vi "Spectrum Interogation routine (SIR).vi"() -> ()   [LabVIEW 2014]
doc: "This is a pretty complex VI probably best to just e-mail me if you need help"
uses:
  Subs/Global 1.vi
  <vilib>/Utility/file.llb/Read From Spreadsheet File (DBL).vi
  <vilib>/measure/mamon.llb/Waveform Peak Detection for 1 Chan.vi
  <vilib>/Utility/file.llb/Write To Spreadsheet File (DBL).vi
  <vilib>/Utility/file.llb/Read From Spreadsheet File (string).vi
  <vilib>/Utility/file.llb/Write To Spreadsheet File (I64).vi
  <vilib>/measure/NI_MAPro.lvlib
  <vilib>/Analysis/NI_AALBase.lvlib
panel:
  out "subarray":dbl[](array[numeric])
  out "Vally pos":sgl[][](array[numeric])
  out "mark":i32[](array[numeric])
  in  "System Save Data Button":bool
  out "Delimit":string
  out "intensities":sgl[][](array[numeric])
  out "First scan":sgl[][](array[numeric])
  out "Important thing L":i32[](array[numeric])
  out "Important thing R":i32[](array[numeric])
  out "Data layout":u16
  out "File style":enum32{"Radio Selection 1", "Radio Selection 2"}(ring)
  out "Crop bottom":dbl
  out "Crop top":i32
  out "Croppped wave":sgl[](array[numeric])
  out "T0":i32
  out "no' length":i32
  in  "stop":bool
  in  "Tab settings":T1(tab)
  in  "Save to file":bool
  in  "Numeric":i32=1
  in  "Type":T2(radio)=enum."Manual scan frequency"
  in  "Ring":i64(ring) items=["hh:mm:ss", "hh mm ss"]
  in  "Output":T3(radio)=enum."Use time since first scan"
  in  "Gap between files":i32=1
  in  "Start file number":i32 min=0
  in  "Filename No' format":u16(ring) items=["full #"]
  in  "End wavelength":dbl=1160.0 min=0.0 max=1039.27001953125 step=1.0
  in  "Start wavelength":dbl=512.0 min=0.0 max=1039.27001953125 step=1.0
  in  "Xcol":i32 caption="X Col" min=-1 step=1
  in  "yCol":i32=1 caption="Y Col" min=0
  in  "Peak\npointyness":sgl=0.1 caption="Pointyness" min=0 step=0.1
  in  "Vally\npointyness":sgl=0.1 min=0 step=0.1
  in  "Poly order":i32=3
  in  "Minium length":i32=10
  in  "EnH choice":u16(ring) items=["Off", "Linear best fit", "Polynomial best fit", "Moving average"]
  in  "Threshold  2":dbl=1000.0 caption="Threshold" format="%.2p"
  in  "Width 2":i32=15 caption="Width" min=3
  in  "Threshold":dbl=4000.0 format="%.2p"
  in  "Width":i32=15 min=3
  in  "Tracking \nTollerance P":i32=5
  in  "Tracking \nTollerance V":i32=5
  in  "Peaks (T/F)":bool=TRUE
  in  "Vallys (T/F)":bool
  in  "% tracking \nerror":sgl=0.5
  in  "% tracking \nerror V":sgl=0.5
  in  "Lower \nthreshold":u16
  in  "Spectrum\nMoving AV":i32=1 min=1 step=1
  in  "Cross location":dbl=765.105
  in  "Norm":bool
  in  "Substract":bool
  in  "Load sub":bool
  in  "Valid Scans":i32=619
  out "first file loc":path
  out "Detecting Peaks":bool
  out "Plotting graph":bool
  out "Scan":i32(slide)=-1 max=1036 scale=-1.0..4.0
  out "Saving Data":bool
  out "Filtering Peaks":bool caption="Finished"
  out "Load indic":bool
  in  "Load":bool
  out "Number of files":i32=620
  in  "Tab Control":T4(tab)=enum."Intensity plot"
  out "Full":T5(graph)
  in  "System Save Data Button 2":bool
  in  "Play as movie":bool
  in  "ms per scan":u32=100
  in  "Scrollbar":i32(c297)
  out "Movie Plot":T6(graph)
  out "Scan Number":i32
  in  "Combo Box":string(combo)
  out "Intensity Graph":dbl[][](graph)
  in  "Axis Settings":bool
  in  "Save Image":bool
  in  "Top":u32(colorbox)
  in  "Bottom":u32(colorbox)=16777215
  out "Mark position":dbl
  in  "Tab Control 2":enum32{"Peak position", "Peak intensity"}(tab)
  out "Peak position vs Trace number":sgl[][](graph)
  out "Peak Intensity vs Trace number":sgl[][](graph)
  out "Number of\npeaks found":i32
  in  "Tab Control 3":enum32{"Vally position", "Vally intensity"}(tab)
  in  "save av stdev":bool
  out "Vally position vs Trace number":sgl[][](graph)=[[1.0], [1.0], [1.0], [1.0], [1.0], [1.0], [1.0], [1.0], [1.0], [1.0], [1.0], [1.0], [1.0], [1.0], [1.0], [1.0], [1.0], [1.0], [1.0], [1.0], [1.0], [1.0], [1.0], [1.0], [1.0], [1.0], [1.0], [1.0], [1.0], [1.0], [1.0], [1.0], [1.0], [1.0], [1.0], [1.0], [1.0], [1.0], [1.0], [1.0], [1.0], [1.0], [1.0], [1.0], [1.0], [1.0], [1.0], [1.0], [1.0], [1.0], [1.0], [1.0], [1.0], [1.0], [1.0], [1.0], [1.0], [1.0], [1.0], [1.0], [1.0], [1.0], [1.0], [1.0], [1.0], [1.0], [1.0], [1.0], [1.0], [1.0], [1.0], [1.0], [1.0], [1.0], [1.0], [1.0], [1.0], [1.0], [1.0], [1.0], [1.0], [1.0], [1.0], [1.0], [1.0], [1.0], [1.0], [1.0], [1.0], [1.0], [1.0], [1.0], [1.0], [1.0], [1.0], [1.0], [1.0], [1.0], [1.0], [1.0], [1.0], [1.0], [1.0], [1.0], [1.0], [1.0], [1.0], [1.0], [1.0], [1.0], [1.0], [1.0], [1.0], [1.0], [1.0], [1.0], [1.0], [1.0], [1.0], [1.0], [1.0], [1.0], [1.0], [1.0], [1.0], [1.0], [1.0], [1.0], [1.0], [1.0], [1.0], [1.0], [1.0], [1.0], [1.0], [1.0], [1.0], [1.0], [1.0], [1.0], [1.0], [1.0], [1.0], [1.0], [1.0], [1.0], [1.0], [1.0], [1.0], [1.0], [1.0], [1.0], [1.0], [1.0], [1.0], [1.0], [1.0], [1.0], [1.0], [1.0], [1.0], [1.0], [1.0], [1.0], [1.0], [1.0], [1.0], [1.0], [1.0], [1.0], [1.0], [1.0], [1.0], [1.0], [1.0], [1.0], [1.0], [1.0], [1.0], [1.0], [1.0], [1.0], [1.0], [1.0], [1.0], [1.0], [1.0], [1.0], [1.0], [1.0], [1.0], [1.0], [1.0], [1.0], [1.0], [1.0], [1.0], [1.0], [1.0], [1.0], [1.0], [1.0], [1.0], [1.0], [1.0], [1.0], [1.0], [1.0], [1.0], [1.0], [1.0], [1.0], [1.0], [1.0], [1.0], [1.0], [1.0], [1.0], [1.0], [1.0], [1.0], [1.0], [1.0], [1.0], [1.0], [1.0], [1.0], [1.0], [1.0], [1.0], [1.0], [1.0], [1.0], [1.0], [1.0], [1.0], [1.0], [1.0], [1.0], [1.0], [1.0], [1.0], [1.0], [1.0], [1.0], [1.0], [1.0], [1.0], [1.0], [1.0], [1.0], [1.0], [1.0], [1.0], [1.0], [1.0], [1.0], [1.0], [1.0], [1.0], [1.0], [1.0], [1.0], [1.0], [1.0], [1.0], [1.0], [1.0], [1.0], [1.0], [1.0], [1.0], [1.0], [1.0], [1.0], [1.0], [1.0], [1.0], [1.0], [1.0], [1.0], [1.0], [1.0], [1.0], [1.0], [1.0], [1.0], [1.0], [1.0], [1.0], [1.0], [1.0], [1.0], [1.0], [1.0], [1.0], [1.0], [1.0], [1.0], [1.0], [1.0], [1.0], [1.0], [1.0], [1.0], [1.0], [1.0], [1.0], [1.0], [1.0], [1.0], [1.0], [1.0], [1.0], [1.0], [1.0], [1.0], [1.0], [1.0], [1.0], [1.0], [1.0], [1.0], [1.0], [1.0], [1.0], [1.0], [1.0], [1.0], [1.0], [1.0], [1.0], [1.0], [1.0], [1.0], [1.0], [1.0], [1.0], [1.0], [1.0], [1.0], [1.0], [1.0], [1.0], [1.0], [1.0], [1.0], [1.0], [1.0], [1.0], [1.0], [1.0], [1.0], [1.0], [1.0], [1.0], [1.0], [1.0], [1.0], [1.0], [1.0], [1.0], [1.0], [1.0], [1.0], [1.0], [1.0], [1.0], [1.0], [1.0], [1.0], [1.0], [1.0], [1.0], [1.0], [1.0], [1.0], [1.0], [1.0], [1.0], [1.0], [1.0], [1.0], [1.0], [1.0], [1.0], [1.0], [1.0], [1.0], [1.0], [1.0], [1.0], [1.0], [1.0], [1.0], [1.0], [1.0], [1.0], [1.0], [1.0], [1.0], [1.0], [1.0], [1.0], [1.0], [1.0], [1.0], [1.0], [1.0], [1.0], [1.0], [1.0], [1.0], [1.0], [1.0], [1.0], [1.0], [1.0], [1.0], [1.0], [1.0], [1.0], [1.0], [1.0], [1.0], [1.0], [1.0], [1.0], [1.0], [1.0], [1.0], [1.0], [1.0], [1.0], [1.0], [1.0], [1.0], [1.0], [1.0], [1.0], [1.0], [1.0], [1.0], [1.0], [1.0], [1.0], [1.0], [1.0], [1.0], [1.0], [1.0], [1.0], [1.0], [1.0], [1.0], [1.0], [1.0], [1.0], [1.0], [1.0], [1.0], [1.0], [1.0], [1.0], [1.0], [1.0], [1.0], [1.0], [1.0], [1.0], [1.0], [1.0], [1.0], [1.0], [1.0], [1.0], [1.0], [1.0], [1.0], [1.0], [1.0], [1.0], [1.0], [1.0], [1.0], [1.0], [1.0], [1.0], [1.0], [1.0], [1.0], [1.0], [1.0], [1.0], [1.0], [1.0], [1.0], [1.0], [1.0], [1.0]]
  in  "Average size":dbl=1.0 min=1.0 step=1.0
  out "Peak average value":dbl[](array[numeric])
  out "Vally Intensity vs Trace number":sgl[][](graph)
  out "Number of\nvallys found":i32
  out "XY Graph":cluster{i32[], "Data AVs":dbl[]}(graph)
  in  "System Start Button":bool
  in  "Slide":dbl(slide) min=597.927001953125 max=1031.6429443359375 step=0.2 scale=597.927001953125..1031.751953125
  in  "Run":bool
  in  "QUIT":bool
  # "Time stamps"
  # "seconds"
  # "Tracking config"
  # "Peaks"
  # "Vallys"
  # "Enhanced tracking"
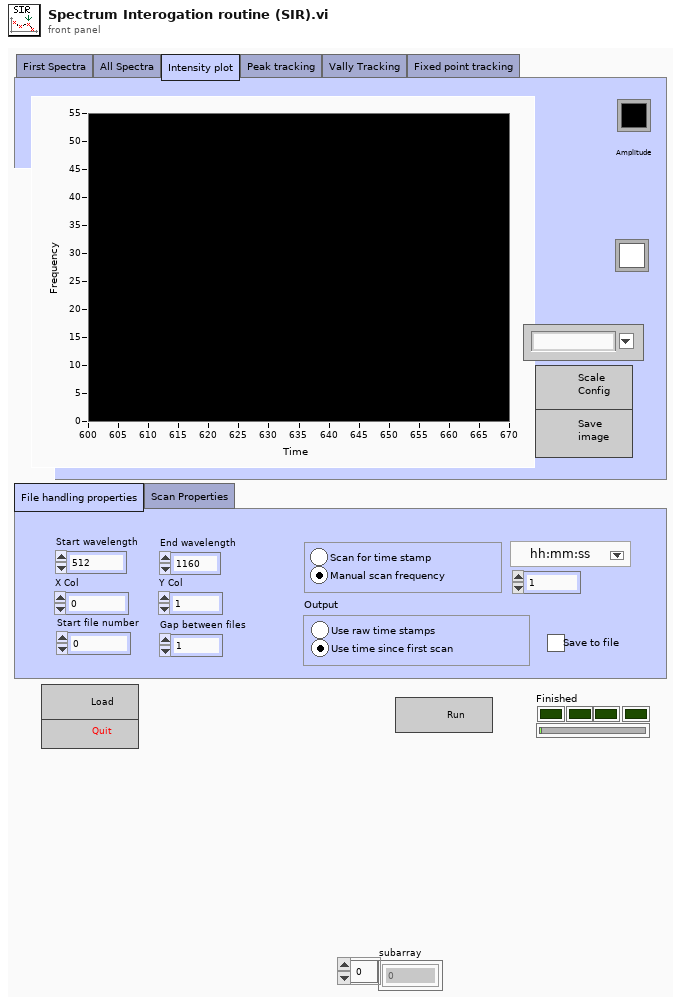
[diagram p1: front panel]
types:
  T1 = enum32{"File handling properties", "Scan Properties"}
  T2 = enum32{"Scan for time stamp", "Manual scan frequency"}
  T3 = enum32{"Use raw time stamps", "Use time since first scan"}
  T4 = enum32{"First Spectra", "All Spectra", "Intensity plot", "Peak tracking", "Vally Tracking", "Fixed point tracking"}
  T5 = cluster{"Feature locations":dbl[], "Intensities":dbl[]}[]
  T6 = cluster{"Croppped wavelengths":sgl[], "Cropped Spectrums":sgl[]}[]
  T7 = enum32{"First Spectra", "All Spectra", "Intensity plot", "Peak tracking", "Vally Tracking"}
  T8 = typedef "imagedata.ctl" = cluster{"image type":i32, "image depth":i32, "image":u8[], "mask":u8[], "colors":u32[], "Rectangle":cluster{"left":i16, "top":i16, "right":i16, "bottom":i16}}
  T9 = cluster{"YScale.Maximum":dbl, "YScale.Minimum":dbl, "YScale.ScaleFit":u8}
  T10 = cluster{"XScale.Maximum":dbl, "XScale.Minimum":dbl, "XScale.ScaleFit":u8}
  T11 = cluster{"ZScale.Maximum":dbl, "ZScale.Minimum":dbl, "ZScale.ScaleFit":u8}
  T12 = cluster{"Vally position vs Trace number":sgl[], "Vally Intensity vs Trace number":sgl[]}
  T13 = cluster{"Peak position vs Trace number":sgl[], sgl[]}
  T14 = cluster{"Croppped wave":sgl[], "intensities":sgl[]}
  T15 = cluster{"Vally position vs Trace number":sgl[], "Vally Intensity vs Trace number":sgl[]}[]
  T16 = cluster{"first file loc":path, "File style":enum32{"Radio Selection 1", "Radio Selection 2"}, "Filename No' format":u16, "Data layout":u16, "Crop top":i32, "Crop bottom":dbl, "Important thing R":i32[], "Important thing L":i32[], "First scan":sgl[][], "Delimit":string}
  T17 = cluster{"Path":path, "File style":enum32{"Radio Selection 1", "Radio Selection 2"}, "Filename No' format ":u16, "Data layout":u16, "Crop top":i32, "Crop bottom":dbl, "Important thing R":i32[], "Important thing L":i32[], sgl[][], "Delimit ":string}
  T18 = cluster{"Feature locations":dbl[], "Intensities":dbl[]}
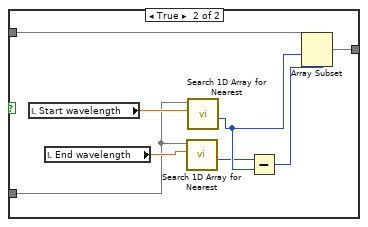
[diagram p4: hidden frame]
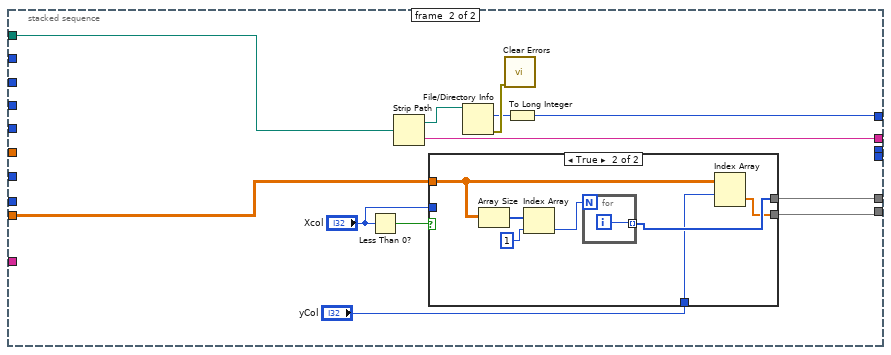
[diagram p7: hidden frame]
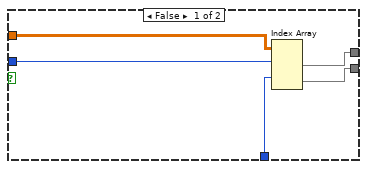
[diagram p8: hidden frame]
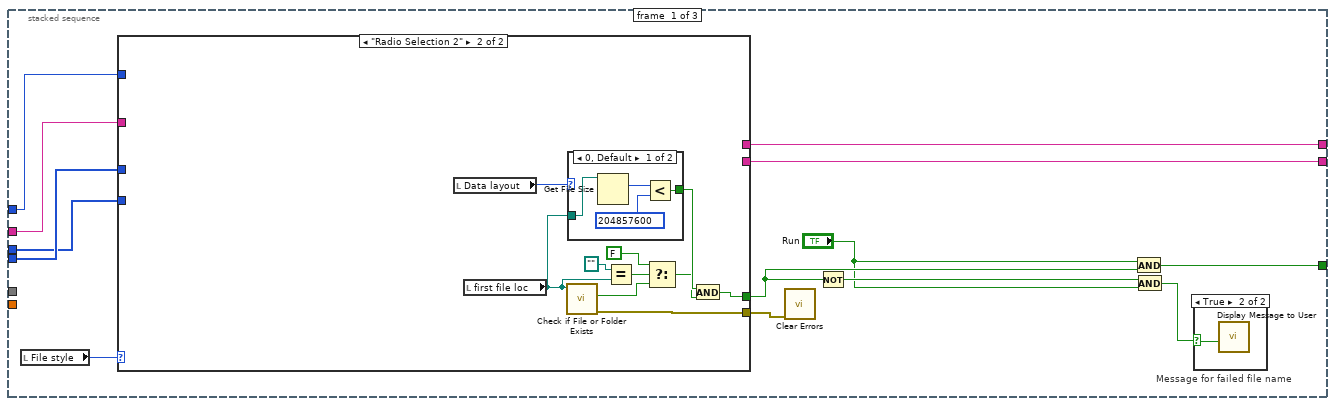
[diagram p9: hidden frame]
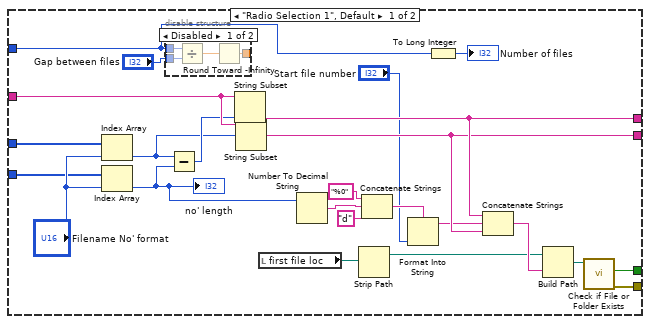
[diagram p10: hidden frame]
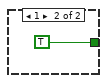
[diagram p12: hidden frame]
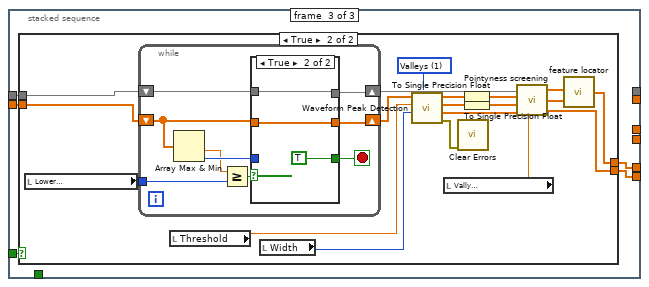
[diagram p19: hidden frame]
diagram:
  w7 = FALSE
  n1 = local write "Tab Control"(T7."First Spectra" ("Tab Control")) -> ()
  n2 = local write "First scan"(sgl[][] []) -> ()
  n3 = local write "first file loc"(path "") -> ()
  n4 = local write "QUIT"(w7) -> ()
  n5 = local write "Saving Data"(w7) -> ()
  n6 = local write "Scan"(-1) -> ()
  n7 = local write "Detecting Peaks"(w7) -> ()
  n8 = local write "Plotting graph"(w7) -> ()
  n9 = local write "Filtering Peaks"(w7) -> ()
  n10 = property on="Plotting graph" class="Bool (strict)"("Blinking"=w7) -> ()  [unwired: 2 in, 2 out]
  n11 = property on="Saving Data" class="Bool (strict)"("Blinking"=w7) -> ()  [unwired: 2 in, 2 out]
  n12 = property on="Filtering Peaks" class="Bool (strict)"("Caption.Text"="Waiting") -> ()  [unwired: 2 in, 2 out]
  n13 = property on="Filtering Peaks" class="Bool (strict)"("Blinking"=w7) -> ()  [unwired: 2 in, 2 out]
  n14 = property on="Detecting Peaks" class="Bool (strict)"("Blinking"=w7) -> ()  [unwired: 2 in, 2 out]
  n15 = local write "stop"(w7) -> ()
  n16 = property on="stop" class="Bool (strict)"("Visible"=w7) -> ()  [unwired: 2 in, 2 out]
  n17 = while {
    shift-right: [w36] -> _
    shift-left: 1 -> [w35]
    stop <- FALSE stop-if-true
    n18 = local read "EnH choice"() -> (w33:u16)
    n19 = local read "Filename No' format"() -> (w27:u16)
    n20 = Wait (ms)(milliseconds to wait=u32 10) -> ()  [unwired: 1 out]
    n21 = local read "Important thing R"() -> (w23:i32[])
    n22 = local read "Important thing L"() -> (w22:i32[])
    n23 = local read "Crop bottom"() -> (w24:dbl)
    n24 = Quit LabVIEW(quit? (T)="QUIT") -> ()
    n25 = local read "first file loc"() -> (w19:path)
    n26 = local read "Data layout"() -> (w26:u16)
    n27 = local read "Delimit"() -> (w17:string)
    n28 = local read "First scan"() -> (w21:sgl[][])
    n29 = local read "Crop top"() -> (w25:i32)
    n30 = local read "File style"() -> (w28:enum32{"Radio Selection 1", "Radio Selection 2"})
    n31 = case "Controls for individual tabs" shown="\"Intensity plot\"" "Tab Control" {
      tunnel: [w322 w324 w384 w390 w402 _] -> w36
      tunnel: w35 -> [w322 w324 w384 w390 w403 _]
      frame "First Spectra", Default {
      }
      frame "Intensity plot" {
        (unwired) u32[] [458778, 589853, 655393, 720933, 852008, 917548, 983087, 1114163, 1179703, 1310778, 1376318, 1441858, 1507397, 1572937, 1572940, 1638480, 1638484, 1704023, 1704027, 1769567, 1769570, 1769574, 1769577, 1835117, 1835121, 1835124, 1835128, 1835132, 1769599, 1769603, 1769606, 1769610, 1704078, 1704081, 1638549, 1638553, 1573020, 1573024, 1507491, 1441959, 1441963, 1376430, 1310898, 1245366, 1179834, 1114307, 1048775, 983243, 917711, 786644, 721116, 655584, 524516, 458984, 327917, 196853, 197113, 66045, 511, 1023, 264703, 528383, 792063, 792063, 1121279, 1384959, 1648639, 1912063, 2241279, 2504703, 2768383, 3031807, 3361023, 3624447, 3887871, 4151295, 4480511, 4743935, 5007359, 5270783, 5533951, 5862911, 6126335, 6389759, 6652927, 6981887, 7245055, 7508479, 7771647, 8100351, 8363775, 8626943, 8890111, 9218815, 9481983, 9745151, 10008063, 10336767, 10599935, 10863103, 11126015, 11454719, 11717631, 11980799, 12243711, 12572159, 12835071, 13098239, 13361151, 13689599, 13952511, 14215167, 14478079, 14806527, 15069439, 15332095, 15595007, 15923199, 16186111, 16448511, 16776958, 16776443, 16775671, 16775155, 16774384, 16773868, 16773096, 16772325, 16771553, 16770781, 16770010, 16769238, 16768466, 16767694, 16766923, 16766151, 16765379, 16764608, 16763580, 16762808, 16762037, 16761009, 16760237, 16759210, 16758438, 16757410, 16756382, 16755611, 16754583, 16753555, 16752528, 16751500, 16750728, 16749701, 16748673, 16747389, 16746362, 16745334, 16744306, 16743278, 16741995, 16740967, 16739939, 16738656, 16737628, 16736344, 16735061, 16734033, 16732749, 16731466, 16730438, 16729154, 16727870, 16726862, 16725835, 16724808, 16724037, 16723010, 16721984, 16721213, 16720186, 16719159, 16718389, 16717362, 16716335, 16715308, 16714538, 16713511, 16712484, 16711714, 16580642, 16580642, 16449570, 16318499, 16187427, 15859747, 15728675, 15597603, 15466531, 15269923, 15007779, 14876708, 14680100, 14549028, 14417956, 14090276, 13959204, 13828132, 13565988, 13369380, 13238308, 13041700, 12845092, 12714020, 12517412, 12320804, 12189731, 11993123, 11796515, 11665443, 11468835, 11272227, 11141155, 10944547, 10747938, 10616866, 10420258, 10223650, 10092578, 9895969, 9699361, 9568289, 9371680, 9175072, 9044000, 8847392, 8650783, 8519711, 8323103, 8126494, 7995422, 7798813, 7602205, 7471133, 7274524, 7077916, 6946843, 6750235, 6553626, 6422554, 6225945, 6029337, 5898264, 5701656, 5505047]  # Color table (Seismic)
        (unwired) u32[] [0, 257, 197379, 1285, 460551, 592137, 2571, 3085, 3599, 3857, 4114, 4628, 4886, 5144, 5402, 5660, 5918, 6176, 6434, 6691, 6693, 6951, 6953, 7211, 7213, 7471, 7473, 7475, 7477, 7478, 7480, 7482, 7484, 7486, 7232, 7491, 7236, 6980, 6469, 6213, 5957, 5702, 5446, 5191, 4935, 4424, 4168, 3912, 3657, 3145, 2890, 2634, 2123, 1867, 1612, 1100, 844, 589, 77, 78, 131150, 196687, 327759, 393295, 393295, 524368, 589904, 720977, 786513, 917586, 983122, 1114195, 1245267, 1310803, 1441876, 1572948, 1638485, 1769557, 1900630, 1966166, 2097238, 2228311, 2359383, 2424920, 2555992, 2687065, 2818137, 2949210, 3080282, 3211354, 3276891, 3473499, 3604572, 3670108, 3866717, 3997790, 4194399, 4325473, 4522082, 4718691, 4915301, 5046374, 5242983, 5439593, 5636202, 5832811, 6029421, 6291566, 6488175, 6684785, 6881394, 7143539, 7340149, 7602294, 7798903, 7929975, 7995510, 8061045, 8192116, 8257651, 8323185, 8454256, 8519791, 8585326, 8716396, 8781931, 8847466, 8978536, 9044071, 9109605, 9175139, 9306210, 9371744, 9437278, 9568349, 9633883, 9699417, 9830487, 9896021, 9961555, 10092625, 10158158, 10223692, 10354762, 10420552, 10486086, 10617156, 10682689, 10748223, 10879292, 10944826, 11010359, 11141428, 11206962, 11272495, 11403564, 11468841, 11534374, 11665443, 11730976, 11796509, 11927578, 11993111, 12189716, 12451857, 12713997, 12976138, 13303815, 13565955, 13830656, 14093824, 14356992, 14685696, 14948864, 15212032, 15344128, 15410688, 15543040, 15609600, 15741696, 15808256, 15940608, 16072961, 16140034, 16272388, 16339461, 16471815, 16538888, 16671498, 16738316, 16739597, 16740879, 16740879, 16742160, 16743442, 16744723, 16746005, 16747031, 16748312, 16749594, 16750619, 16751901, 16752926, 16753952, 16755233, 16756259, 16757285, 16758310, 16759592, 16760617, 16761643, 16762668, 16763438, 16764463, 16765489, 16766515, 16767541, 16768568, 16769597, 16770626, 16771656, 16772429, 16773458, 16774232, 16775005, 16775778, 16776295, 16777069, 16711538, 16514935, 16383868, 16252802, 16187271, 16056204, 15990673, 15925143, 15859612, 15794081, 15728551, 15728556, 15728561, 15728566, 15728572, 15728577, 15728582, 15794123, 15859665, 15925206, 15990747, 16056288, 16187366, 16252907, 16383984, 16515062, 16646139, 11184809]  # Color table (Space)
        (unwired) u32[] [16777215, 16777213, 16711675, 16646137, 16646135, 16580597, 16580595, 16515057, 16515055, 16449517, 16449515, 16449513, 16449511, 16449509, 16449507, 16449505, 16449503, 16449501, 16449499, 16449497, 16515031, 16515029, 16515027, 16580561, 16646095, 16646093, 16711627, 16777161, 16777159, 16777157, 16776899, 16776641, 16776383, 16776125, 16775867, 16775353, 16775095, 16774837, 16774323, 16774065, 16773551, 16773293, 16772778, 16772264, 16772006, 16771492, 16770978, 16770464, 16769950, 16769436, 16768922, 16768152, 16767638, 16767124, 16766610, 16765840, 16765326, 16764556, 16763786, 16763272, 16762502, 16761732, 16760962, 16760448, 16760448, 16759678, 16758908, 16757882, 16757112, 16756342, 16755572, 16754802, 16753776, 16753006, 16751980, 16751210, 16750184, 16749158, 16748388, 16747362, 16746336, 16745310, 16744284, 16743258, 16742232, 16741206, 16739923, 16738897, 16737871, 16736589, 16735563, 16734281, 16733255, 16731973, 16730691, 16729665, 16728127, 16727612, 16726592, 16726337, 16725827, 16725317, 16724807, 16724297, 16723788, 16723278, 16722768, 16722259, 16721749, 16721240, 16720731, 16720222, 16719713, 16719203, 16718695, 16718186, 16717677, 16717168, 16716660, 16716151, 16715643, 16715134, 16714626, 16714118, 16713609, 16713101, 16712593, 16712086, 16646298, 16515229, 16384161, 16253092, 16122024, 15990955, 15859887, 15728818, 15597749, 15466680, 15335611, 15204542, 15073473, 14942404, 14811334, 14680265, 14549195, 14418126, 14287056, 14155986, 14024917, 13697236, 13304018, 12910800, 12517582, 12124364, 11731146, 11337928, 11010246, 10617028, 10289346, 9896128, 9568446, 9240764, 8913082, 8585400, 8257718, 7930036, 7602354, 7274672, 6946990, 6684844, 6357162, 6095015, 5767333, 5505187, 5243041, 4980895, 4718749, 4456603, 4194457, 3932311, 3670165, 3473555, 3211409, 3014799, 2752653, 2556043, 2359433, 2162823, 1900677, 1704067, 1507457, 1376383, 1376383, 1179773, 983163, 786553, 852087, 458869, 327795, 196721, 65647, 109, 875, 1385, 1639, 2149, 3427, 3169, 3423, 3933, 4187, 4697, 4951, 5205, 5458, 5712, 5966, 6220, 6474, 6728, 6726, 6980, 6978, 7232, 7230, 7228, 7482, 7480, 7478, 7476, 7474, 7216, 7214, 7212, 6954, 6952, 6694, 6436, 6434, 6176, 5918, 5660, 5402, 5144, 4630, 4372, 4114, 3600, 3342, 2828, 2317, 2056, 1542, 1027, 131072, 0]  # Color table (Saturn)
        (unwired) u32[] [3538998, 3801146, 4128830, 4390978, 4587590, 4784201, 5046349, 5242960, 5439571, 5701719, 5898330, 6094941, 6357089, 6553700, 6815848, 7012459, 7209070, 7471218, 7667829, 7864440, 8126588, 8323199, 8519807, 8716415, 8978559, 9175167, 9371775, 9568383, 9764991, 10027135, 10223743, 10420351, 10616959, 10813567, 11010175, 11272319, 11468927, 11665535, 11862143, 12058751, 12320895, 12517503, 12714111, 12910719, 13107327, 13369471, 13566079, 13762687, 13959295, 14155903, 14352511, 14614655, 14811263, 15007871, 15204479, 15401087, 15663231, 15859839, 16056447, 16253055, 16449663, 16711807, 16712578, 16713349, 16713349, 16714121, 16714892, 16715663, 16716690, 16717461, 16718233, 16719004, 16719775, 16720802, 16721573, 16722344, 16723116, 16723887, 16724914, 16725685, 16726456, 16727228, 16727999, 16728770, 16729797, 16730568, 16731340, 16732111, 16732882, 16733909, 16734680, 16735451, 16736223, 16736994, 16738021, 16738792, 16739563, 16740335, 16741106, 16741877, 16742904, 16743675, 16744447, 16744703, 16744959, 16744959, 16745215, 16745471, 16745727, 16745983, 16746239, 16746239, 16746495, 16746751, 16747007, 16747263, 16747519, 16747519, 16747775, 16748031, 16748287, 16748543, 16748799, 16748799, 16749055, 16749311, 16749567, 16749823, 16750079, 16750079, 16750335, 16750591, 16750847, 16751103, 16751103, 16751359, 16751615, 16751871, 16752127, 16752383, 16752383, 16752639, 16752895, 16753151, 16753407, 16753663, 16753663, 16753919, 16754175, 16754431, 16754687, 16754943, 16754943, 16755199, 16755455, 16755711, 16755967, 16756223, 16756223, 16756479, 16756735, 16756991, 16757247, 16757503, 16757503, 16757759, 16758015, 16758271, 16758527, 16758527, 16758783, 16759039, 16759295, 16759551, 16759807, 16759807, 16760063, 16760319, 16760575, 16760831, 16761087, 16761087, 16761343, 16761599, 16761855, 16762111, 16762367, 16762367, 16762623, 16762879, 16763135, 16763391, 16763391, 16763647, 16763647, 16763903, 16764159, 16764415, 16764671, 16764671, 16764927, 16765183, 16765439, 16765695, 16765951, 16765951, 16766207, 16766463, 16766719, 16766975, 16767231, 16767231, 16767487, 16767743, 16767999, 16768255, 16768511, 16768511, 16768767, 16769023, 16769279, 16769535, 16769791, 16769791, 16770047, 16770303, 16770559, 16770815, 16770815, 16771071, 16771327, 16771583, 16771839, 16772095, 16772095, 16772351, 16772607, 16772863, 16773119, 16773375, 16773375, 16773631, 16773887, 16774143, 16774399, 16774655, 16774655, 16774911, 16775167, 16775423, 16775679, 16775935, 16775935, 16776191, 16776447, 16776703]  # Color table (Rose)
        (unwired) u32[] [162896, 227667, 292437, 357208, 421979, 487005, 551776, 616547, 877926, 746089, 811115, 875886, 940657, 1070964, 1135991, 1200761, 1265532, 1330303, 1395330, 1460100, 1524871, 1589898, 1654668, 1719439, 1784465, 1849236, 1914262, 1979033, 2109595, 2174366, 2239136, 2304162, 2369189, 2433959, 2498985, 2563755, 2628781, 2693807, 2758577, 2823603, 2888629, 2953654, 3018424, 3148985, 3214779, 3279036, 3344062, 3409087, 3474112, 3539138, 3604931, 3670980, 3737029, 3803077, 3869126, 3935687, 4000967, 4132552, 4198600, 4264393, 4330441, 4396233, 4462281, 4528074, 4528074, 4594121, 4659913, 4725961, 4791753, 4857544, 4923592, 4989383, 5055175, 5186502, 5252293, 5318085, 5383876, 5449667, 5515458, 5581248, 5647039, 5712830, 5778364, 5844155, 5909945, 5975480, 6041270, 6107061, 6238131, 6303665, 6369455, 6434989, 6500779, 6566313, 6631847, 6697381, 6762914, 6828448, 6893982, 6959515, 7025049, 7090582, 7221652, 7287185, 7352719, 7418252, 7483530, 7549063, 7614340, 7679874, 7745407, 7810684, 7875961, 7941495, 8006772, 8072049, 8137582, 8268395, 8333673, 8398950, 8464227, 8529504, 8594781, 8660059, 8725336, 8790613, 8855891, 8920912, 8986189, 9051466, 9116744, 9181765, 9312579, 9377600, 9442878, 9507899, 9573177, 9638198, 9703220, 9768498, 9833520, 9899310, 9963563, 10028841, 10093863, 10158885, 10223907, 10354722, 10420768, 10486814, 10552861, 10618907, 10685721, 10751000, 10817303, 10883349, 10949396, 11015443, 11081746, 11147793, 11213840, 11345679, 11411727, 11477774, 11544077, 11610125, 11676428, 11742476, 11808780, 11874828, 11941132, 12007180, 12073484, 12139788, 12205836, 12272140, 12403981, 12470029, 12536334, 12602638, 12668687, 12734992, 12801297, 12867602, 12933651, 12999956, 13066261, 13132566, 13198616, 13264921, 13331226, 13463068, 13463068, 13529374, 13595423, 13661729, 13728035, 13794341, 13860647, 13926953, 13993003, 14059309, 14125615, 14191921, 14258227, 14324278, 14456120, 14522426, 14588733, 14655039, 14721090, 14787396, 14853703, 14920010, 14986060, 15052367, 15118674, 15184980, 15251031, 15317338, 15383645, 15515231, 15581538, 15647589, 15713896, 15780202, 15846253, 15912560, 15978611, 16044918, 16110968, 16177275, 16243326, 16309377, 16375683, 16441734, 16573577, 16639627, 16705678, 16771729, 16706963, 16641942, 16576920, 16511899, 16446877, 16381855, 16316834, 16251812, 16186790, 16121768, 15990186, 15924140, 15858094, 15792048, 15726002, 15660212]  # Color table (Morning glory)
        (unwired) u32[] [3355443, 2697513, 1842204, 921102, 328965, 131586, 460551, 1184274, 2171169, 3223857, 3947580, 4276545, 4079166, 3421236, 2565927, 1644825, 1052688, 855309, 1184274, 1907997, 2894892, 3947580, 4671303, 5000268, 4802889, 4144959, 3289650, 2368548, 1776411, 1579032, 1842204, 2631720, 3618615, 4671303, 5395026, 5723991, 5526612, 4934475, 4013373, 3092271, 2500134, 2302755, 2565927, 3355443, 4342338, 5395026, 6118749, 6447714, 6250335, 5592405, 4737096, 3815994, 3223857, 3026478, 3289650, 4079166, 5066061, 6118749, 6842472, 7171437, 6974058, 6316128, 5460819, 4539717, 4539717, 3947580, 3750201, 4013373, 4802889, 5789784, 6842472, 7566195, 7895160, 7697781, 7039851, 6184542, 5263440, 4671303, 4473924, 4737096, 5526612, 6513507, 7566195, 8289918, 8618883, 8421504, 7763574, 6908265, 5987163, 5395026, 5197647, 5460819, 6250335, 7237230, 8289918, 9013641, 9342606, 9145227, 8487297, 7631988, 6710886, 6118749, 5921370, 6184542, 6974058, 7960953, 9013641, 9737364, 10066329, 9868950, 9211020, 8355711, 7434609, 6842472, 6579300, 6908265, 7697781, 8684676, 9671571, 10461087, 10790052, 10592673, 9934743, 9079434, 8158332, 7500402, 7303023, 7631988, 8421504, 9408399, 10395294, 11184810, 11513775, 11316396, 10658466, 9803157, 8882055, 8224125, 8026746, 8355711, 9145227, 10132122, 11119017, 11908533, 12237498, 12040119, 11382189, 10526880, 9605778, 8947848, 8750469, 9079434, 9868950, 10855845, 11842740, 12632256, 12961221, 12763842, 12105912, 11250603, 10329501, 9671571, 9474192, 9803157, 10592673, 11579568, 12566463, 13355979, 13684944, 13487565, 12829635, 11974326, 11053224, 10395294, 10197915, 10526880, 11316396, 12303291, 13290186, 14079702, 14408667, 14211288, 13553358, 12632256, 11776947, 11119017, 10921638, 11250603, 11974326, 13027014, 14013909, 14803425, 14803425, 15132390, 14935011, 14277081, 13355979, 12500670, 11842740, 11645361, 11974326, 12698049, 13750737, 14737632, 15527148, 15856113, 15658734, 15000804, 14079702, 13224393, 12566463, 12369084, 12698049, 13421772, 14474460, 15461355, 16250871, 16579836, 16382457, 15724527, 14803425, 13948116, 13290186, 13092807, 13421772, 14145495, 15198183, 16185078, 16645629, 16316664, 16514043, 16448250, 15527148, 14671839, 14013909, 13816530, 14145495, 14869218, 15921906, 16711422, 15921906, 15592941, 15790320, 16448250, 16250871, 15395562, 14737632, 14540253, 14869218, 15592941, 16645629, 15987699, 15198183, 14935011, 15066597, 15724527]  # Color table (GrayScale-banded)
        n32 = case "Exports intensity graph as image" shown="True" "Save Image" {
          frame False {
          }
          frame True {
            n33 = invoke on="Intensity Graph" class="IntGraph (strict)" method="Get Image"("image depth"=24 ("Image Depth")) -> (error out=w372:errorcluster, "image data"=w373:T8)  [unwired: 5 in, 4 out]
            n34 = local write "Save Image"(FALSE) -> ()
            n35 = call "File Dialog2"() -> ("selected path"=w374:path, "error out"=w371:errorcluster)  [unwired: 12 in, 2 out]
            n36 = call <vilib>:"Clear Errors.vi"("error in (no error)"=w372) -> ()  [unwired: 5 in, 2 out]
            n37 = case shown="No Error" w371 {
              tunnel: w374 -> [w382 _]
              tunnel: w373 -> [w376 _]
              frame No Error {
                n38 = Strip Path(path=w382) -> (stripped path=w378:path, name=w380:string)
                n39 = Concatenate Strings(w380, ".jpg") -> (w379:string)
                n40 = Build Path(base path=w378, name or relative path=w379) -> (appended path=w377:path)
                n41 = call <vilib>:"Write JPEG File.vi"("quality (80)"=100, "image data"=w376, "path to JPEG file"=w377) -> ()  [unwired: 7 in, 2 out]
              }
              frame Error {
              }
            }
          }
        }
        n42 = case shown="True" "Axis Settings" {
          tunnel: w324 -> [_ _]
          frame False {
          }
          frame True {
            n43 = stacked-sequence {
              tunnel: [_ w362 _] -> w342
              tunnel: [w358 _ _] -> w343
              tunnel: [_ _ w366] -> w341
              frame #0 {
                n44 = property on="Intensity Graph" class="IntGraph (strict)"() -> ("YScale.Maximum"=w361:dbl, "YScale.Minimum"=w360:dbl, "YScale.ScaleFit"=w359:u8)  [unwired: 2 in, 2 out]
                n45 = Bundle("YScale.Maximum"=w361, "YScale.Minimum"=w360, "YScale.ScaleFit"=w359) -> (w358:T9)  [unwired: 1 in]
              }
              frame #1 {
                n46 = property on="Intensity Graph" class="IntGraph (strict)"() -> ("XScale.Maximum"=w365:dbl, "XScale.Minimum"=w364:dbl, "XScale.ScaleFit"=w363:u8)  [unwired: 2 in, 2 out]
                n47 = Bundle("XScale.Maximum"=w365, "XScale.Minimum"=w364, "XScale.ScaleFit"=w363) -> (w362:T10)  [unwired: 1 in]
              }
              frame #2 {
                n48 = property on="Intensity Graph" class="IntGraph (strict)"() -> ("ZScale.Maximum"=w369:dbl, "ZScale.Minimum"=w368:dbl, "ZScale.ScaleFit"=w367:u8)  [unwired: 2 in, 2 out]
                n49 = Bundle("ZScale.Maximum"=w369, "ZScale.Minimum"=w368, "ZScale.ScaleFit"=w367) -> (w366:T11)  [unwired: 1 in]
              }
            }
            n50 = local write "Axis Settings"(FALSE) -> ()
            n51 = call "3d axis settings.vi"("Int Current"=w341, "Wave Current"=w342, "Scan Current"=w343) -> ("Int setting"=w339:T11, "Wave setting"=w340:T11, "Scan setting"=w344:T11)
            n52 = stacked-sequence {
              tunnel: w339 -> [_ _ w355]
              tunnel: w344 -> [w346 _ _]
              tunnel: w340 -> [_ w351 _]
              frame #0 {
                n53 = Unbundle(w346) -> ("ZScale.Maximum"=w349:dbl, "ZScale.Minimum"=w348:dbl, "ZScale.ScaleFit"=w347:u8)
                n54 = property on="Intensity Graph" class="IntGraph (strict)"("YScale.Maximum"=w349, "YScale.Minimum"=w348, "YScale.ScaleFit"=w347) -> ()  [unwired: 2 in, 2 out]
              }
              frame #1 {
                n55 = Unbundle(w351) -> ("ZScale.Maximum"=w353:dbl, "ZScale.Minimum"=w350:dbl, "ZScale.ScaleFit"=w352:u8)
                n56 = property on="Intensity Graph" class="IntGraph (strict)"("XScale.Maximum"=w353, "XScale.Minimum"=w350, "XScale.ScaleFit"=w352) -> ()  [unwired: 2 in, 2 out]
              }
              frame #2 {
                n57 = Unbundle(w355) -> ("ZScale.Maximum"=w357:dbl, "ZScale.Minimum"=w354:dbl, "ZScale.ScaleFit"=w356:u8)
                n58 = property on="Intensity Graph" class="IntGraph (strict)"("ZScale.Maximum"=w357, "ZScale.Minimum"=w354, "ZScale.ScaleFit"=w356) -> ()  [unwired: 2 in, 2 out]
              }
            }
          }
        }
        n59 = case shown="\"Carnation\"" "Combo Box" {
          frame "Carnation" {
            w327 = u32[] [16711691, 16711954, 16712217, 16712480, 16712742, 16713005, 16713268, 16713530, 16713793, 16714056, 16715086, 16714580, 16714842, 16715104, 16715367, 16715629, 16715891, 16716153, 16716415, 16716677, 16716940, 16717202, 16717463, 16717725, 16717987, 16718249, 16718511, 16718772, 16719034, 16719296, 16719557, 16719819, 16720079, 16720341, 16720602, 16720863, 16721125, 16721386, 16721647, 16721908, 16722169, 16722430, 16395007, 16133119, 15805695, 15478271, 15216383, 14888959, 14561535, 14234111, 13972223, 13644799, 13382911, 13055487, 12793599, 12531711, 12269823, 11942399, 11680511, 11418623, 11156735, 10829311, 10567423, 10305535, 10305535, 10043647, 9781503, 9585151, 9323263, 9061375, 8799487, 8537599, 8341247, 8079359, 7883007, 7621119, 7424767, 7228415, 6966527, 6770175, 6573823, 6377471, 6115583, 5919231, 5722879, 5526527, 5527551, 5594111, 5660927, 5727743, 5794559, 5861375, 5927935, 5994751, 6061567, 6128127, 6194943, 6261503, 6328063, 6394879, 6461439, 6527999, 6594815, 6661375, 6727935, 6794495, 6861055, 6927871, 6994175, 7060735, 7127295, 7193855, 7260415, 7326719, 7393279, 7459839, 7526143, 7592703, 7659007, 7725311, 7791871, 7858175, 7924479, 7991039, 8057343, 8123647, 8189951, 8256255, 8322815, 8388605, 8454139, 8519672, 8585205, 8650738, 8716271, 8781804, 8847338, 8912871, 8978404, 9043938, 9109472, 9175005, 9240539, 9306073, 9371606, 9437140, 9502674, 9568208, 9633742, 9699275, 9764809, 9830343, 9895877, 9961412, 10026946, 10092480, 10158014, 10223548, 10289083, 10354617, 10420152, 10485686, 10551221, 10616755, 10682290, 10747825, 10813359, 10878894, 10944429, 11009964, 11075499, 11141034, 11206570, 11403179, 11599788, 11796397, 11993006, 12124079, 12320688, 12517297, 12648370, 12844979, 13041588, 13172661, 13303734, 13500343, 13631416, 13762489, 13959098, 14090171, 14221244, 14352317, 14352317, 14483390, 14614463, 14745535, 14876608, 15007681, 15138754, 15269827, 15335364, 15466437, 15597510, 15663047, 15794120, 15859657, 15990730, 16056267, 16121804, 16252877, 16318414, 16383951, 16515024, 16580561, 16646098, 16711635, 16776916, 16776917, 16776662, 16776407, 16776152, 16775897, 16775642, 16775643, 16775388, 16775133, 16775134, 16775135, 16774880, 16774881, 16774626, 16774627, 16774628, 16774373, 16774374, 16774375, 16774376, 16774377, 16774378, 16774379, 16774380, 16774381, 16774638, 16774639, 16774640, 16774641, 16774898, 16774899, 16775156, 16775157, 16775414, 16775415, 16775672, 16775929, 16776186, 16776187]  # Color table (Carnation)
            n60 = property on="Intensity Graph" class="IntGraph (strict)"("Color Table"=w327) -> ()  [unwired: 2 in, 2 out]
          }
          frame "Hot metal" {
            w328 = u32[] [3407872, 131072, 196608, 327680, 458752, 589824, 655360, 786432, 917504, 1048576, 1114112, 1245184, 1376256, 1507328, 1572864, 1703936, 1835008, 1966080, 2031616, 2162688, 2293760, 2424832, 2555904, 2621440, 2752512, 2883584, 3014656, 3080192, 3211264, 3342336, 3473408, 3538944, 3670016, 3801088, 3932160, 3997696, 4128768, 4259840, 4390912, 4456448, 4587520, 4718592, 4849664, 4980736, 5046272, 5177344, 5308416, 5439488, 5505024, 5636096, 5767168, 5898240, 5963776, 6094848, 6225920, 6356992, 6422528, 6553600, 6684672, 6815744, 6881280, 7012352, 7143424, 7143424, 7274496, 7405568, 7471104, 7602176, 7733248, 7864320, 7929856, 8060928, 8192000, 8323072, 8388608, 8519680, 8650752, 8781824, 8847360, 8978432, 9109504, 9240576, 9306112, 9437184, 9568256, 9699328, 9830400, 9895936, 10027008, 10158080, 10289152, 10354688, 10485760, 10616832, 10747904, 10813440, 10944512, 11075584, 11206656, 11272192, 11403264, 11534336, 11665408, 11730944, 11862016, 11993088, 12124160, 12189696, 12320768, 12451840, 12582912, 12713984, 12779520, 12910592, 13041664, 13172736, 13238272, 13369344, 13500416, 13631488, 13697024, 13828096, 13959168, 14090240, 14155776, 14286848, 14417920, 14548992, 14614528, 14745600, 14876672, 15007744, 15138816, 15204352, 15335424, 15466496, 15597568, 15663104, 15794176, 15925248, 16056320, 16121856, 16252928, 16384000, 16515072, 16580608, 16580608, 16580608, 16515072, 16711680, 16711680, 16711680, 16712192, 16647424, 16713728, 16714496, 16715264, 16716032, 16716800, 16717568, 16718336, 16719104, 16719872, 16720640, 16721408, 16722176, 16722944, 16723712, 16724480, 16725248, 16726016, 16726784, 16727552, 16728064, 16728832, 16729600, 16730368, 16731136, 16731904, 16732672, 16733440, 16734208, 16734976, 16735744, 16736512, 16737280, 16738048, 16738816, 16739584, 16740352, 16741120, 16741120, 16741888, 16742656, 16743424, 16743936, 16744704, 16745472, 16746240, 16747008, 16747776, 16748544, 16749312, 16750080, 16750848, 16751616, 16752384, 16753152, 16753920, 16754688, 16755456, 16756224, 16756992, 16757760, 16758528, 16759296, 16760064, 16760576, 16761344, 16762112, 16762880, 16763648, 16764416, 16765184, 16765952, 16766720, 16767488, 16768256, 16769024, 16769792, 16770560, 16771328, 16772096, 16772864, 16773632, 16774400, 16775168, 16775936, 16776448, 16776960, 16776960, 16776960, 16776960, 16776960, 16776960, 16776960, 16776960, 16776960, 16776960, 16776960, 16776960, 16776960, 16776960, 16776960, 16776448]  # Color table (Hot metal)
            n61 = property on="Intensity Graph" class="IntGraph (strict)"("Color Table"=w328) -> ()  [unwired: 2 in, 2 out]
          }
          frame "Rainbow-striped" {
            w329 = u32[] [12255418, 12386492, 12517567, 12320960, 12189888, 12058817, 11927746, 11731139, 11600067, 9175197, 9044125, 11141318, 11010246, 10813639, 10682568, 10551497, 10354890, 10223818, 10092747, 7930019, 7798948, 9633997, 9502926, 9306319, 9175248, 9044176, 8847569, 8716498, 8585427, 6750377, 6619306, 8126677, 7995606, 7798999, 7667927, 7536856, 7340249, 7209178, 7078106, 5505199, 5374128, 6619357, 6488285, 6291678, 6160607, 6029536, 5832929, 5701857, 5570786, 4325557, 4194486, 5112036, 4980965, 4784358, 4653287, 4522215, 4325608, 4194537, 4063466, 3080380, 3014844, 3604716, 3408109, 3277038, 3277038, 3145966, 3014895, 2818288, 2687217, 2556145, 1900738, 1769666, 2097396, 1900789, 1769717, 1638646, 1507575, 1310968, 1179896, 1048825, 721096, 590024, 590075, 393468, 262397, 131326, 255, 1791, 3327, 4863, 5068, 6348, 9471, 11007, 12543, 14079, 15615, 17151, 18687, 20223, 17612, 18636, 25087, 26623, 28159, 29695, 31231, 32767, 34303, 35839, 29900, 31180, 40447, 41983, 43775, 45311, 46847, 48383, 49919, 51455, 42444, 43724, 56063, 57599, 59135, 60671, 62207, 63743, 65535, 65528, 52418, 52413, 65510, 65504, 65498, 65492, 65486, 65480, 65474, 65468, 52369, 52364, 65449, 65443, 65437, 65431, 65425, 65419, 65413, 65407, 52321, 52316, 65389, 65383, 65377, 65371, 65364, 65358, 65352, 65346, 52272, 52267, 65328, 65322, 65316, 65310, 65304, 65298, 65292, 65286, 52224, 314368, 851712, 1244928, 1638144, 2031360, 2424576, 2817792, 3211008, 3604224, 3197952, 3525632, 4783872, 5177088, 5635840, 6029056, 6422272, 6815488, 7208704, 7601920, 6409216, 6736896, 6736896, 8781568, 9174784, 9568000, 9961216, 10354432, 10747648, 11206400, 11599616, 9554944, 9882624, 12779264, 13172480, 13565696, 13958912, 14352128, 14745344, 15138560, 15531776, 12766208, 13093888, 16776960, 16775170, 16773637, 16771847, 16770314, 16768780, 16766991, 16765457, 13411088, 13409810, 16760601, 16758812, 16757278, 16755745, 16753955, 16752422, 16750888, 16749099, 13398052, 13396774, 16744243, 16742704, 16741166, 16739884, 16738345, 16736807, 16735269, 16733730, 13385753, 13384728, 16729371, 16727833, 16726295, 16725012, 16723474, 16721936, 16720397, 16718859, 13373959, 13372677, 16714500, 16712962, 16711680]  # Color table (Rainbow-striped)
            n62 = property on="Intensity Graph" class="IntGraph (strict)"("Color Table"=w329) -> ()  [unwired: 2 in, 2 out]
          }
          frame "Single colour", Default {
            n63 = property on="Intensity Graph" class="IntGraph (strict)"() -> ("ZScale.Maximum"=w331:dbl, "ZScale.Minimum"=w333:dbl)  [unwired: 2 in, 2 out]
            n64 = Build Array(w331, "Top") -> (w334:dbl[])
            n65 = Build Array(w333, "Bottom") -> (w335:dbl[])
            n66 = Array To Cluster(array=w334) -> (cluster=w337:cluster{"[0]":dbl, "[1]":dbl})
            n67 = Array To Cluster(array=w335) -> (cluster=w336:cluster{"[0]":dbl, "[1]":dbl})
            n68 = Build Array(w337, w336) -> (w338:cluster{"[0]":dbl, "[1]":dbl}[])
            n69 = property on="Intensity Graph" class="IntGraph (strict)"("ZScale.MarkerVals[]"=w338) -> ()  [unwired: 2 in, 2 out]
          }
        }
      }
      frame "Peak tracking" {
      }
      frame "Vally Tracking" {
        n70 = local read "Vally pos"() -> (w389:sgl[][])
        n71 = for {
          tunnel: [w394] -> w388 mode=indexing
          tunnel: w389 -> [w397] mode=indexing
          tunnel: [w393] -> w387 mode=indexing
          n72 = property on="Vally position vs Trace number" class="WFGraph (strict)"() -> ("Cursor.Cursor X"=w399:dbl)  [unwired: 2 in, 2 out]
          n73 = Divide(x="Average size", y=2) -> (x/y=w400:dbl)
          n74 = Add(x=w399, y=w400) -> (x+y=w396:dbl)
          n75 = Delete From Array(array=w397, length="Average size", index=w396) -> (deleted portion=w395:sgl[])  [unwired: 1 out]
          n76 = call <vilib>:"Std Deviation and Variance.vi"("X"=w395) -> ("mean"=w394:dbl, "standard deviation"=w393:dbl)  [unwired: 1 in, 1 out]
        }
        "Peak average value" <- w388
        n77 = Build Array(w388, w387) -> (w386:dbl[][])
        n78 = case shown="True" "save av stdev" {
          tunnel: w386 -> [_ w392]
          frame False {
          }
          frame True {
            n79 = call-poly <vilib>:"Write To Spreadsheet File.vi"("transpose? (no:F)"=TRUE, "2D data"=w392) -> ()  [unwired: 6 in, 1 out]
          }
        }
      }
      frame "All Spectra" {
        n80 = stacked-sequence {
          tunnel: w403 -> [w409 _]
          tunnel: ["Scrollbar" _] -> w402
          frame #0 {
            n81 = local read "Vally Intensity vs Trace number"() -> (w405:sgl[][])
            n82 = local read "Peak Intensity vs Trace number"() -> (w406:sgl[][])
            n83 = local read "Vally position vs Trace number"() -> (w404:sgl[][])
            n84 = local read "Peak position vs Trace number"() -> (w407:sgl[][])
            n85 = local read "Start file number"() -> (w413:i32)
            n86 = local read "Valid Scans"() -> (w412:i32)
            n87 = Not Equal?(x="Scrollbar", y=w409) -> (x != y?=w410:bool)
            n88 = Add(x=w412, y=w413) -> (x+y=w414:i32)
            n89 = case "Plots peak locations on Spectra plot" shown="True" w410 {
              tunnel: "Scrollbar" -> [_ w427]
              tunnel: w407 -> [_ w422]
              tunnel: w406 -> [_ w421]
              tunnel: w404 -> [_ w420]
              tunnel: w405 -> [_ w419]
              frame False {
              }
              frame True {
                n90 = local read "Croppped wave"() -> (w423:sgl[])
                n91 = local read "intensities"() -> (w416:sgl[][])
                n92 = Transpose 2D Array(2D array=w421) -> (transposed array=w424:sgl[][])
                n93 = Index Array(array=w416, index (row)=w427) -> (element=w436:sgl[])  [unwired: 1 in]
                n94 = Index Array(array=w419, index (row)=w427) -> (element=w426:sgl[])  [unwired: 1 in]
                n95 = Index Array(array=w424, index (row)=w427) -> (element=w434:sgl[])  [unwired: 1 in]
                n96 = Index Array(array=w422, index (col)=w427) -> (element=w435:sgl[])  [unwired: 1 in]
                n97 = Index Array(array=w420, index (col)=w427) -> (element=w425:sgl[])  [unwired: 1 in]
                n98 = Bundle("Vally position vs Trace number"=w425, "Vally Intensity vs Trace number"=w426) -> (w417:T12)  [unwired: 1 in]
                n99 = Bundle("Peak position vs Trace number"=w435, w434) -> (w433:T13)  [unwired: 1 in]
                n100 = Bundle("Croppped wave"=w423, "intensities"=w436) -> (w418:T14)  [unwired: 1 in]
                n101 = Array Max & Min(array=w416) -> (max value=w415:sgl)  [unwired: 3 out]
                n102 = Build Array(w418, w433, w417) -> (→"Movie Plot":T15)
                n103 = local read "Gap between files"() -> (w430:i32)
                n104 = disable-structure shown="Disabled" {
                  disable-tunnel: w415 -> [w437 _]
                  frame Disabled {
                    n105 = property on="Movie Plot" class="XYGraph (strict)"("YScale.Maximum"=w437) -> ()  [unwired: 2 in, 2 out]
                  }
                  frame Enabled {
                  }
                }
                n106 = local read "Start file number"() -> (w429:i32)
                n107 = Multiply(x=w427, y=w430) -> (x*y=w431:i32)
                n108 = Add(x=w429, y=w431) -> (x+y=→"Scan Number":i32)
              }
            }
            n109 = case "Animates spectra plots" shown="True" "Play as movie" {
              tunnel: w414 -> [_ w444]
              tunnel: w407 -> [_ w441]
              tunnel: w406 -> [_ w440]
              tunnel: w404 -> [_ w439]
              tunnel: w405 -> [_ w438]
              frame False {
              }
              frame True {
                n110 = while {
                  tunnel: w444 -> [w474]
                  tunnel: [w458] -> w442
                  tunnel: w441 -> [w453]
                  tunnel: w440 -> [w452]
                  tunnel: w439 -> [w451]
                  tunnel: w438 -> [w450]
                  stop <- w458 stop-if-true
                  n111 = local read "Gap between files"() -> (w468:i32)
                  n112 = local read "Scrollbar"() -> (w466:i32)
                  n113 = local read "Play as movie"() -> (w472:bool)
                  n114 = To Long Integer(number=w466) -> (32bit integer=w445:i32)
                  n115 = Add(x=w468, y=w466) -> (x+y=w469:i32)
                  n116 = Add(x=w468, y=w469) -> (x+y=w470:i32)
                  n117 = Not(x=w472) -> (.not. x?=w473:bool)
                  n118 = Greater Or Equal?(x=w470, y=w474) -> (x >= y?=w471:bool)
                  n119 = Or(x=w471, y=w473) -> (x .or. y?=w458:bool)
                  n120 = case shown="False" w471 {
                    tunnel: w469 -> [w476 _]
                    frame False {
                      n121 = local write "Scrollbar"(w476) -> ()
                    }
                    frame True {
                    }
                  }
                  n122 = local read "Croppped wave"() -> (w454:sgl[])
                  n123 = local read "intensities"() -> (w447:sgl[][])
                  n124 = Transpose 2D Array(2D array=w452) -> (transposed array=w455:sgl[][])
                  n125 = Index Array(array=w447, index (row)=w445) -> (element=w446:sgl[])  [unwired: 1 in]
                  n126 = Index Array(array=w455, index (row)=w445) -> (element=w465:sgl[])  [unwired: 1 in]
                  n127 = Index Array(array=w453, index (col)=w445) -> (element=w464:sgl[])  [unwired: 1 in]
                  n128 = Index Array(array=w450, index (row)=w445) -> (element=w456:sgl[])  [unwired: 1 in]
                  n129 = Index Array(array=w451, index (col)=w445) -> (element=w457:sgl[])  [unwired: 1 in]
                  n130 = Bundle("Peak position vs Trace number"=w464, w465) -> (w463:T13)  [unwired: 1 in]
                  n131 = Bundle("Croppped wave"=w454, "intensities"=w446) -> (w448:T14)  [unwired: 1 in]
                  n132 = Bundle("Vally position vs Trace number"=w457, "Vally Intensity vs Trace number"=w456) -> (w449:T12)  [unwired: 1 in]
                  n133 = Build Array(w448, w463, w449) -> (w467:T15)
                  n134 = local write "Movie Plot"(w467) -> ()
                  n135 = local read "Gap between files"() -> (w459:i32)
                  n136 = Multiply(x=w445, y=w459) -> (x*y=w460:i32)
                  n137 = local read "Start file number"() -> (w461:i32)
                  n138 = Add(x=w461, y=w460) -> (x+y=w462:i32)
                  n139 = Wait (ms)(milliseconds to wait="ms per scan") -> ()  [unwired: 1 out]
                  n140 = local write "Scan Number"(w462) -> ()
                }
                n141 = Not(x=w442) -> (.not. x?=w443:bool)
                n142 = local write "Play as movie"(w443) -> ()
              }
            }
          }
          frame #1 {
            n143 = First Call?() -> (First Call?: T/F=w477:bool)
            n144 = case shown="True" w477 {
              frame False {
              }
              frame True {
                n145 = for {
                  tunnel: i32[] [0, 1, 2] -> [w488] mode=indexing
                  tunnel: i32[] [2, 0, 0] -> [w487] mode=indexing
                  tunnel: i32[] [0, 1, 1] -> [w486] mode=indexing
                  tunnel: i32[] [0, 4, 4] -> [w485] mode=indexing
                  tunnel: [w484] -> w479 mode=indexing
                  n146 = property on="Movie Plot" class="XYGraph (strict)"("Active Plot"=w488, "Plot.Plot Interpolation"=w487, "Plot.Point Style"=w486, "Plot.Line Width"=w485) -> (error out=w484:errorcluster)  [unwired: 2 in, 1 out]
                }
                n147 = Merge Errors(w479) -> (w478:errorcluster)
                n148 = call <vilib>:"Clear Errors.vi"("error in (no error)"=w478) -> ()  [unwired: 5 in, 2 out]
              }
            }
          }
        }
      }
      frame "Fixed point tracking" {
        n149 = local read "Start wavelength"() -> (w489:dbl)
        n150 = local read "End wavelength"() -> (w490:dbl)
        n151 = local read "Croppped wave"() -> (w494:sgl[])
        n152 = property on="Slide" class="Slide (strict)"("Scale.Maximum"=w490, "Scale.Minimum"=w489) -> ()  [unwired: 2 in, 2 out]
        n153 = Array Max & Min(array=w494) -> (max value=w493:sgl, min value=w492:sgl)  [unwired: 2 out]
        n154 = property on="Slide" class="Slide (strict)"("Maximum"=w493, "Minimum"=w492) -> ()  [unwired: 2 in, 2 out]
        n155 = case shown="True" TRUE {
          tunnel: "Slide" -> [_ w505]
          tunnel: w494 -> [_ w504]
          frame False {
          }
          frame True {
            n156 = local read "intensities"() -> (w502:sgl[][])
            n157 = call "Search 1D Array for Nearest.vi"("desired element"=w505, "1D Array"=w504) -> ("closest index"=w501:i32, "closest element"=w503:dbl)  [unwired: 8 in]
            n158 = local write "Slide"(w503) -> ()
            n159 = local read "Spectrum\nMoving AV"() -> (w496:i32)
            n160 = for {
              tunnel: w502 -> [w509] mode=indexing
              tunnel: w501 -> [w513]
              tunnel: [w512] -> w497 mode=indexing
              tunnel: [w511] -> w499 mode=indexing
              tunnel: w496 -> [w508]
              i -> [w511]
              n161 = call "Moving average.vi"("Width of AV"=w508, "Raw data"=w509) -> ("Data AVs"=w510:dbl[])  [unwired: 1 in, 1 out]
              n162 = Index Array(array=w510, index=w513) -> (element=w512:dbl)
            }
            n163 = case shown="True" "System Start Button" {
              tunnel: w497 -> [_ w507]
              frame False {
              }
              frame True {
                n164 = call-poly <vilib>:"Write To Spreadsheet File.vi"("transpose? (no:F)"=TRUE, "1D data"=w507) -> ()  [unwired: 6 in, 1 out]
              }
            }
            n165 = Bundle(w499, w497) -> (→"XY Graph":cluster{i32[], dbl[]})  [unwired: 1 in]
          }
        }
      }
    }
    n166 = Equal?(x=w33, y=2) -> (x = y?=w31:bool)
    n167 = property on="Poly order" class="DigNum (strict)"("Visible"=w31) -> ()  [unwired: 2 in, 2 out]
    n168 = case shown="True" "Load" {
      frame False {
      }
      frame True {
        n169 = local write "Load"(FALSE) -> ()
        "Load indic" <- TRUE
      }
    }
    n170 = stacked-sequence {
      tunnel: [w83 _] -> w18
      tunnel: [w82 _] -> w16
      tunnel: w28 -> [w81 _]
      tunnel: w27 -> [w80 _]
      tunnel: w26 -> [w79 _]
      tunnel: w25 -> [w78 _]
      tunnel: w24 -> [w77 _]
      tunnel: w23 -> [w76 _]
      tunnel: w22 -> [w75 _]
      tunnel: w19 -> [w74 w120]
      tunnel: w21 -> [w73 w116]
      tunnel: [_ w122] -> w41
      tunnel: [_ w121] -> w20
      tunnel: [_ w119] -> w15
      tunnel: [_ w118] -> w12
      tunnel: w17 -> [w72 _]
      frame #0 {
        n171 = local read "Load indic"() -> (w84:bool)
        n172 = case "Loading new data set into program" shown="True" w84 {
          tunnel: [w85 w91] -> w82
          tunnel: [w86 w92] -> w83
          tunnel: w74 -> [_ w106]
          tunnel: w81 -> [_ w105]
          tunnel: w80 -> [_ w104]
          tunnel: w79 -> [_ w103]
          tunnel: w78 -> [_ w102]
          tunnel: w77 -> [_ w101]
          tunnel: w76 -> [w86 w100]
          tunnel: w75 -> [w85 w99]
          tunnel: w73 -> [_ w98]
          tunnel: w72 -> [_ w89]
          frame False {
          }
          frame True {
            n173 = local write "Load indic"(FALSE) -> ()
            n174 = Bundle("first file loc"=w106, "File style"=w105, "Filename No' format"=w104, "Data layout"=w103, "Crop top"=w102, "Crop bottom"=w101, "Important thing R"=w100, "Important thing L"=w99, "First scan"=w98, "Delimit"=w89) -> (w110:T16)  [unwired: 1 in]
            n175 = call "Advanced file handeling.vi"("Data in"=w110) -> ("File out"=w113:T17)  [unwired: 4 in]
            n176 = local read "Xcol"() -> (w88:i32)
            n177 = Unbundle(w113) -> ("Path"=→"first file loc":path, "File style"=→"File style":enum32{"Radio Selection 1", "Radio Selection 2"}, "Filename No' format"=w108:u16, "Data layout"=→"Data layout":u16, "Crop top"=→"Crop top":i32, "Crop bottom"=→"Crop bottom":dbl, "Important thing R"=w92:i32[], "Important thing L"=w91:i32[], w95:sgl[][], "Delimit"=→"Delimit":string)
            "Important thing R" <- w92
            "Important thing L" <- w91
            "First scan" <- w95
            n178 = Index Array(array=w95, index (row)=w88) -> (element=w87:sgl[])  [unwired: 1 in]
            n179 = Array Max & Min(array=w87) -> (max value=w94:sgl, min value=w93:sgl)  [unwired: 2 out]
            n180 = local write "Filename No' format"(w108) -> ()
            n181 = local write "End wavelength"(w94) -> ()
            n182 = local write "Start wavelength"(w93) -> ()
            n183 = property on="Full" class="XYGraph (strict)"("XScale.Maximum"=w94, "XScale.Minimum"=w93) -> ()  [unwired: 2 in, 2 out]
            n184 = property on="Start wavelength" class="DigNum (strict)"("Maximum"=w94, "Minimum"=w93) -> ()  [unwired: 2 in, 2 out]
            n185 = property on="End wavelength" class="DigNum (strict)"("Maximum"=w94, "Minimum"=w93) -> ()  [unwired: 2 in, 2 out]
          }
        }
      }
      frame #1 {
        n186 = Less Than 0?(x="Xcol") -> (x < 0?=w115:bool)
        n187 = Strip Path(path=w120) -> (stripped path=w123:path, name=w121:string)
        n188 = case shown="True" w115 {
          tunnel: [w130 w134] -> w119
          tunnel: [w129 w132] -> w118
          tunnel: "yCol" -> [w128 w133]
          tunnel: w116 -> [w127 w137]
          tunnel: "Xcol" -> [w126 _]
          frame False {
            n189 = Index Array(array=w127, index (row) #1=w126, index (row) #2=w128) -> (element #1=w130:sgl[], element #2=w129:sgl[])  [unwired: 2 in]
          }
          frame True {
            n190 = Array Size(array=w137) -> (size(s)=w136:i32[])
            n191 = Index Array(array=w136, index=1) -> (element=w135:i32)
            n192 = for {
              N: w135 -> [_]
              tunnel: [w138] -> w134 mode=indexing
              i -> [w138]
            }
            n193 = Index Array(array=w137, index (row)=w133) -> (element=w132:sgl[])  [unwired: 1 in]
          }
        }
        n194 = File/Directory Info(path=w123) -> (size=w124:i64, error out=w125:errorcluster)  [unwired: 1 in, 5 out]
        n195 = call <vilib>:"Clear Errors.vi"("error in (no error)"=w125) -> ()  [unwired: 5 in, 2 out]
        n196 = To Long Integer(number=w124) -> (32bit integer=w122:i32)
      }
    }
    n197 = local read "Xcol"() -> (w8:i32)
    n198 = local read "yCol"() -> (w9:i32)
    n199 = global write "Global 1.vi" "yCol"(w9) -> ()
    n200 = global write "Global 1.vi" "xCol"(w8) -> ()
    n201 = local read "Substract"() -> (w10:bool)
    n202 = case shown="True" "Load sub" {
      tunnel: w9 -> [_ w55]
      tunnel: w8 -> [_ w51]
      frame False {
      }
      frame True {
        n203 = call-poly <vilib>:"Read From Spreadsheet File.vi"() -> ("all rows"=w54:dbl[][])  [unwired: 7 in, 4 out]
        n204 = local write "Load sub"(FALSE) -> ()
        n205 = local read "Norm"() -> (w48:bool)
        n206 = Index Array(array=w54, index (col) #1=w55, index (col) #2=w51) -> (element #1=w53:dbl[], element #2=w50:dbl[])  [unwired: 2 in]
        n207 = case shown="True" w48 {
          tunnel: w53 -> [w66 w68]
          tunnel: [w66 w67] -> w52
          frame False {
          }
          frame True {
            n208 = Array Max & Min(array=w68) -> (max value=w71:dbl)  [unwired: 3 out]
            n209 = Divide(x=100, y=w71) -> (x/y=w69:dbl)
            n210 = Multiply(x=w69, y=w68) -> (x*y=w67:dbl[])
          }
        }
        n211 = case shown="False" w48 {
          tunnel: w52 -> [w57 w60]
          tunnel: w50 -> [_ w59]
          tunnel: [w57 w58] -> w49
          frame False {
          }
          frame True {
            n212 = local read "Start wavelength"() -> (w61:dbl)
            n213 = local read "End wavelength"() -> (w62:dbl)
            n214 = call "Search 1D Array for Nearest.vi"("desired element"=w62, "1D Array"=w59) -> ("closest index"=w63:i32)  [unwired: 8 in, 1 out]
            n215 = call "Search 1D Array for Nearest.vi"("desired element"=w61, "1D Array"=w59) -> ("closest index"=w64:i32)  [unwired: 8 in, 1 out]
            n216 = Subtract(x=w63, y=w64) -> (x-y=w65:i32)
            n217 = Array Subset(array=w60, index=w64, length=w65) -> (w58:dbl[])
          }
        }
        "subarray" <- w49
      }
    }
    n218 = case shown="True" w10 {
      tunnel: w12 -> [w42 w45]
      tunnel: [w42 w43] -> w11
      frame False {
      }
      frame True {
        n219 = local read "subarray"() -> (w44:dbl[])
        n220 = Divide(x=w45, y=w44) -> (x/y=w46:dbl[])
        n221 = Multiply(x=w46, y=100) -> (x*y=w43:dbl[])
      }
    }
    n222 = stacked-sequence {
      tunnel: w20 -> [w144 _ _]
      tunnel: [w147 _ _] -> w30
      tunnel: [w146 _ _] -> w14
      tunnel: [w139 _ _] -> w29
      tunnel: w41 -> [w145 _ _]
      tunnel: w11 -> [_ w204 _]
      tunnel: w15 -> [_ w207 _]
      tunnel: w16 -> [w142 _ _]
      tunnel: w18 -> [w141 _ _]
      frame #0 {
        n223 = local read "File style"() -> (w140:enum32{"Radio Selection 1", "Radio Selection 2"})
        n224 = case shown="\"Radio Selection 2\"" w140 {
          tunnel: [w175 w187] -> w151
          tunnel: [w174 w189] -> w148
          tunnel: [w171 _] -> w147
          tunnel: [w170 _] -> w146
          tunnel: w145 -> [w152 _]
          tunnel: w144 -> [w169 _]
          tunnel: w142 -> [w157 _]
          tunnel: w141 -> [w156 _]
          frame "Radio Selection 1", Default {
            n225 = Index Array(array=w157, index="Filename No' format") -> (element=w166:i32)
            n226 = Index Array(array=w156, index="Filename No' format") -> (element=w161:i32)
            "no' length" <- w161
            n227 = disable-structure shown="Disabled" {
              disable-tunnel: "Gap between files" -> [w178 _]
              disable-tunnel: w152 -> [w177 _]
              disable-tunnel: [w176 _] -> _
              frame Disabled {
                n228 = Divide(x=w177, y=w178) -> (x/y=w179:dbl)
                n229 = Round Toward -Infinity(1:w179) -> (0:w176:dbl)
              }
              frame Enabled {
              }
            }
            n230 = Subtract(x=w166, y=w161) -> (x-y=w167:i32)
            n231 = String Subset(string=w169, length (rest)=w167) -> (substring=w171:string)  [unwired: 1 in]
            n232 = String Subset(string=w169, offset (0)=w166) -> (substring=w170:string)  [unwired: 1 in]
            n233 = local read "first file loc"() -> (w155:path)
            n234 = Number To Decimal String(number=w161) -> (decimal integer string=w163:string)  [unwired: 1 in]
            n235 = Strip Path(path=w155) -> (stripped path=w154:path)  [unwired: 1 out]
            n236 = Concatenate Strings("%0", w163, "d") -> (w165:string)
            n237 = Format Into String(format string=w165, "Start file number") -> (resulting string=w159:string)  [unwired: 2 in, 1 out]
            n238 = To Long Integer(number=w152) -> (32bit integer=→"Number of files":i32)
            n239 = Concatenate Strings(w171, w159, w170) -> (w172:string)
            n240 = Build Path(base path=w154, name or relative path=w172) -> (appended path=w173:path)
            n241 = call <vilib>:"Check if File or Folder Exists.vi"("path"=w173) -> ("error out"=w174:errorcluster, "file or folder exists?"=w175:bool)  [unwired: 8 in, 1 out]
          }
          frame "Radio Selection 2" {
            n242 = local read "Data layout"() -> (w186:u16)
            n243 = local read "first file loc"() -> (w184:path)
            n244 = call <vilib>:"Check if File or Folder Exists.vi"("path"=w184) -> ("error out"=w189:errorcluster, "file or folder exists?"=w181:bool)  [unwired: 8 in, 1 out]
            n245 = case shown="0, Default" w186 {
              tunnel: w184 -> [w193 _]
              tunnel: [w190 TRUE] -> w188
              frame 0, Default {
                n246 = Get File Size(file=w193) -> (size (in bytes)=w191:i64)  [unwired: 1 in, 2 out]
                n247 = Less?(x=w191, y=204857600) -> (x < y?=w190:bool)
              }
              frame 1 {
              }
            }
            n248 = Equal?(x=path "", y=w184) -> (x = y?=w185:bool)
            n249 = Select(t=FALSE, s=w185, f=w181) -> (s? t:f=w180:bool)
            n250 = And(x=w188, y=w180) -> (x .and. y?=w187:bool)
          }
        }
        n251 = call <vilib>:"Clear Errors.vi"("error in (no error)"=w148) -> ()  [unwired: 5 in, 2 out]
        n252 = Not(x=w151) -> (.not. x?=w150:bool)
        n253 = And(x="Run", y=w151) -> (x .and. y?=w139:bool)
        n254 = And(x=w150, y="Run") -> (x .and. y?=w149:bool)
        n255 = case "Message for failed file name" shown="True" w149 {
          selector: w149 -> [_ w195]
          frame False {
          }
          frame True {
            n256 = call "Display Message to User"("Enable"=w195) -> ()  [unwired: 9 in, 2 out]
          }
        }
      }
      frame #1 {
        n257 = Array Size(array=w204) -> (size(s)=w208:i32)
        n258 = call "Moving average.vi"("Width of AV"="Spectrum\nMoving AV", "Raw data"=w204) -> ("Data AVs"=w206:dbl[])  [unwired: 1 in, 1 out]
        n259 = Equal To 0?(x=w208) -> (x = 0?=w209:bool)
        n260 = case shown="False" w209 {
          tunnel: w207 -> [w233 _]
          tunnel: w206 -> [w223 _]
          tunnel: [w232 _] -> w197
          tunnel: [w231 _] -> w196
          tunnel: [w230 _] -> w200
          tunnel: [w229 _] -> w199
          tunnel: [w228 _] -> w202
          tunnel: [w227 _] -> w201
          frame False {
            n261 = local read "Norm"() -> (w224:bool)
            n262 = local read "Peaks (T/F)"() -> (w226:bool)
            n263 = case shown="True" w224 {
              tunnel: w223 -> [w234 w236]
              tunnel: [w234 w235] -> w222
              frame False {
              }
              frame True {
                n264 = Array Max & Min(array=w236) -> (max value=w239:dbl)  [unwired: 3 out]
                n265 = Divide(x=100, y=w239) -> (x/y=w237:dbl)
                n266 = Multiply(x=w237, y=w236) -> (x*y=w235:dbl[])
              }
            }
            n267 = local read "Vallys (T/F)"() -> (w225:bool)
            n268 = stacked-sequence {
              tunnel: w233 -> [w243 w262 w265]
              tunnel: w222 -> [w244 w261 w264]
              tunnel: [w241 _ _] -> w230
              tunnel: [w242 _ _] -> w229
              tunnel: [_ _ w267] -> w231
              tunnel: [_ _ w266] -> w232
              tunnel: [_ w262 _] -> w228
              tunnel: [_ w261 _] -> w227
              tunnel: w226 -> [w240 _ _]
              tunnel: w225 -> [_ _ w263]
              frame #0 {
                n269 = case shown="True" w240 {
                  tunnel: w244 -> [_ w259]
                  tunnel: w243 -> [_ w251]
                  tunnel: [_ w250] -> w242
                  tunnel: [_ w249] -> w241
                  frame False {
                  }
                  frame True {
                    w260 = u16 0 items=["Peaks", "Valleys"] ("peaks/valleys")
                    n270 = local read "Threshold  2"() -> (w248:dbl)
                    n271 = local read "Width 2"() -> (w247:i32)
                    n272 = local read "Peak\npointyness"() -> (w246:sgl)
                    n273 = call-poly <vilib>:"Waveform Peak Detection.vi"("peaks/valleys"=w260, "width"=w247, "threshold"=w248, "Signal In"=w259) -> ("error out"=w245:errorcluster, "2nd Derivatives"=w252:dbl[], "Amplitudes"=w253:dbl[], "Locations"=w254:dbl[])  [unwired: 3 in, 1 out]
                    n274 = call <vilib>:"Clear Errors.vi"("error in (no error)"=w245) -> ()  [unwired: 5 in, 2 out]
                    n275 = To Single Precision Float(number=w254) -> (single precision float=w255:sgl[])
                    n276 = To Single Precision Float(number=w253) -> (single precision float=w257:sgl[])
                    n277 = call "Pointyness screening.vi"("Scan Loc"=w251, "Feature Loc"=w255, "Intensities"=w257, "Peak\npointyness"=w246, "2nd Derivatives"=w252) -> ("Scan Loc"=w258:dbl[], "Feature Loc"=w256:dbl[], "Intensities"=w249:dbl[])  [unwired: 1 in]
                    n278 = call "feature locator.vi"("Features"=w256, "Locations"=w258) -> ("Feature locations"=w250:dbl[])
                  }
                }
              }
              frame #1 {
              }
              frame #2 {
                n279 = case shown="True" w263 {
                  tunnel: [_ w279] -> w267
                  tunnel: [_ w278] -> w266
                  tunnel: w265 -> [_ w277]
                  tunnel: w264 -> [_ w276]
                  frame False {
                  }
                  frame True {
                    w273 = u16 1 items=["Peaks", "Valleys"] ("peaks/valleys")
                    n280 = local read "Lower \nthreshold"() -> (w269:u16)
                    n281 = while {
                      tunnel: w269 -> [w288]
                      shift-right: [w292] -> w274
                      shift-left: w276 -> [w293]
                      shift-right: [w289] -> w275
                      shift-left: w277 -> [w290]
                      stop <- w294 stop-if-true
                      n282 = Array Max & Min(array=w293) -> (min value=w287:dbl, min index (indices)=w291:i32)  [unwired: 2 out]
                      n283 = Greater Or Equal?(x=w287, y=w288) -> (x >= y?=w295:bool)
                      n284 = case shown="True" w295 {
                        tunnel: [FALSE TRUE] -> w294
                        tunnel: w293 -> [w300 w302]
                        tunnel: [w299 w302] -> w292
                        tunnel: w291 -> [w296 _]
                        tunnel: w290 -> [w298 w303]
                        tunnel: [w297 w303] -> w289
                        frame False {
                          n285 = Delete From Array(array=w298, index=w296) -> (array with subset deleted=w297:sgl[])  [unwired: 1 in, 1 out]
                          n286 = Delete From Array(array=w300, index=w296) -> (array with subset deleted=w299:dbl[])  [unwired: 1 in, 1 out]
                        }
                        frame True {
                        }
                      }
                    }
                    n287 = local read "Threshold"() -> (w272:dbl)
                    n288 = local read "Width"() -> (w271:i32)
                    n289 = call-poly <vilib>:"Waveform Peak Detection.vi"("peaks/valleys"=w273, "width"=w271, "threshold"=w272, "Signal In"=w274) -> ("error out"=w268:errorcluster, "2nd Derivatives"=w280:dbl[], "Amplitudes"=w281:dbl[], "Locations"=w282:dbl[])  [unwired: 3 in, 1 out]
                    n290 = local read "Vally\npointyness"() -> (w270:sgl)
                    n291 = call <vilib>:"Clear Errors.vi"("error in (no error)"=w268) -> ()  [unwired: 5 in, 2 out]
                    n292 = To Single Precision Float(number=w282) -> (single precision float=w283:sgl[])
                    n293 = To Single Precision Float(number=w281) -> (single precision float=w285:sgl[])
                    n294 = call "Pointyness screening.vi"("Scan Loc"=w275, "Feature Loc"=w283, "Intensities"=w285, "Peak\npointyness"=w270, "2nd Derivatives"=w280) -> ("Scan Loc"=w286:dbl[], "Feature Loc"=w284:dbl[], "Intensities"=w279:dbl[])  [unwired: 1 in]
                    n295 = call "feature locator.vi"("Features"=w284, "Locations"=w286) -> ("Feature locations"=w278:dbl[])
                  }
                }
              }
            }
          }
          frame True {
          }
        }
        n296 = Bundle("First scan"=w202, "Data AVs"=w201) -> (w213:cluster{"First scan":sgl[], "Data AVs":dbl[]})  [unwired: 1 in]
        n297 = Bundle("Feature locations"=w199, "Intensities"=w200) -> (w212:T18)  [unwired: 1 in]
        n298 = Bundle("Feature locations"=w197, "Intensities"=w196) -> (w211:T18)  [unwired: 1 in]
        n299 = case "Save scan as it" shown="True" "System Save Data Button" {
          tunnel: w201 -> [_ w220]
          tunnel: w202 -> [_ w219]
          frame False {
          }
          frame True {
            n300 = Build Array(w219, w220) -> (w221:dbl[][])
            n301 = call-poly <vilib>:"Write To Spreadsheet File.vi"("transpose? (no:F)"=TRUE, "2D data"=w221) -> ()  [unwired: 6 in, 1 out]
          }
        }
        n302 = case "Save vallys as it" shown="True" "System Save Data Button 2" {
          tunnel: w196 -> [_ w216]
          tunnel: w197 -> [_ w215]
          frame False {
          }
          frame True {
            n303 = Build Array(w215, w216) -> (w217:dbl[][])
            n304 = call-poly <vilib>:"Write To Spreadsheet File.vi"("transpose? (no:F)"=TRUE, "2D data"=w217) -> ()  [unwired: 6 in, 1 out]
          }
        }
        n305 = Build Array(w213, w212, w211) -> (→"Full":T5)
      }
      frame #2 {
        n306 = First Call?() -> (First Call?: T/F=w305:bool)
        n307 = stacked-sequence {
          frame #0 {
            n308 = local read "Threshold  2"() -> (w307:dbl)
            n309 = property on="Full" class="XYGraph (strict)"("Active Cursor"=u32 0, "Cursor.Cursor Y"=w307) -> ()  [unwired: 2 in, 2 out]
          }
          frame #1 {
            n310 = local read "Threshold"() -> (w308:dbl)
            n311 = property on="Full" class="XYGraph (strict)"("Active Cursor"=u32 1, "Cursor.Cursor Y"=w308) -> ()  [unwired: 2 in, 2 out]
          }
          frame #2 {
            n312 = local read "Start wavelength"() -> (w310:dbl)
            n313 = property on="Full" class="XYGraph (strict)"("Active Cursor"=u32 2, "Cursor.Cursor X"=w310) -> ()  [unwired: 2 in, 2 out]
          }
          frame #3 {
            n314 = local read "End wavelength"() -> (w312:dbl)
            n315 = property on="Full" class="XYGraph (strict)"("Active Cursor"=u32 3, "Cursor.Cursor X"=w312) -> ()  [unwired: 2 in, 2 out]
          }
        }
        n316 = case shown="True" w305 {
          frame False {
          }
          frame True {
            n317 = for {
              tunnel: i32[] [0, 1, 2] -> [w321] mode=indexing
              tunnel: i32[] [2, 0, 0] -> [w320] mode=indexing
              tunnel: i32[] [0, 1, 1] -> [w319] mode=indexing
              tunnel: i32[] [0, 4, 4] -> [w318] mode=indexing
              n318 = property on="Full" class="XYGraph (strict)"("Active Plot"=w321, "Plot.Plot Interpolation"=w320, "Plot.Point Style"=w319, "Plot.Line Width"=w318) -> ()  [unwired: 2 in, 2 out]
            }
          }
        }
      }
    }
    n319 = case "Peak dectection and plotting routiens" shown="True" w29 {
      tunnel: w30 -> [w545 _]
      tunnel: w14 -> [w544 _]
      frame True {
        w539 = FALSE
        n320 = local write "Filtering Peaks"(w539) -> ()
        n321 = local write "Saving Data"(w539) -> ()
        n322 = local write "Plotting graph"(w539) -> ()
        n323 = local write "Detecting Peaks"(w539) -> ()
        n324 = local write "Valid Scans"(0) -> ()
        n325 = local read "first file loc"() -> (w517:path)
        n326 = local read "File style"() -> (w520:enum32{"Radio Selection 1", "Radio Selection 2"})
        n327 = flat-sequence {
          tunnel: w517 -> [w552]
          tunnel: w544 -> [w553]
          tunnel: w545 -> [w554]
          tunnel: [w551] -> w532
          tunnel: w520 -> [w550]
          tunnel: [w547] -> w519
          tunnel: [w546] -> w518
          tunnel: [w640] -> w538
          tunnel: [w639] -> w536
          tunnel: w532 -> [w644]
          tunnel: [w624] -> w530
          tunnel: [w642] -> w528
          tunnel: [w641] -> w527
          tunnel: [w636] -> w526
          tunnel: [w635] -> w525
          tunnel: w519 -> [w631]
          tunnel: w518 -> [w632]
          tunnel: w538 -> [w935]
          tunnel: [w932] -> w537
          tunnel: w536 -> [w934]
          tunnel: [w933] -> w535
          tunnel: [w929] -> w534
          tunnel: [w928] -> w533
          tunnel: w530 -> [w936]
          tunnel: [w936] -> w529
          tunnel: w528 -> [w931]
          tunnel: w527 -> [w930]
          tunnel: w526 -> [w927]
          tunnel: w525 -> [w926]
          tunnel: [w927] -> w524
          tunnel: [w926] -> w523
          tunnel: w537 -> [w1029]
          tunnel: w535 -> [w1028]
          tunnel: w534 -> [w1027]
          tunnel: w533 -> [w1024]
          tunnel: [w1029] -> w543
          tunnel: [w1028] -> w542
          tunnel: [w1024] -> w541
          tunnel: [w1027] -> w540
          tunnel: w529 -> [w1030]
          tunnel: w524 -> [w1026]
          tunnel: w523 -> [w1025]
          tunnel: [w1026] -> w522
          tunnel: [w1025] -> w521
          tunnel: w543 -> [w1102]
          tunnel: w542 -> [w1100]
          tunnel: w541 -> [w1101]
          tunnel: w540 -> [w1103]
          tunnel: w522 -> [w1089]
          tunnel: w521 -> [w1093]
          tunnel: [w1086] -> w516
          tunnel: w516 -> [w1174]
          frame #0 {
            n328 = local read "Gap between files"() -> (w549:i32)
            n329 = local read "Start file number"() -> (w548:i32)
            n330 = case shown="\"Radio Selection 1\", Default" w550 {
              selector: w550 -> [w555 w592]
              tunnel: w554 -> [w562 _]
              tunnel: w553 -> [w561 _]
              tunnel: w552 -> [w560 w585]
              tunnel: [w559 _] -> w551
              tunnel: w549 -> [w557 w591]
              tunnel: w548 -> [w556 w590]
              tunnel: [_ w593] -> w547
              tunnel: [w555 w592] -> w546
              frame "Radio Selection 1", Default {
                n331 = local read "Number of files"() -> (w558:i32)
                n332 = for "Checks for the number of valid scan files in the  directory" {
                  N: w558 -> [_]
                  tunnel: w562 -> [w580]
                  tunnel: w561 -> [w575]
                  tunnel: w560 -> [w563]
                  tunnel: [w576] -> w559 mode=indexing
                  tunnel: w557 -> [w566]
                  tunnel: w556 -> [w565]
                  i -> [w582]
                  n333 = local read "no' length"() -> (w569:i32)
                  n334 = Number To Decimal String(number=w569) -> (decimal integer string=w570:string)  [unwired: 1 in]
                  n335 = Multiply(x=w566, y=w582) -> (x*y=w581:i32)
                  n336 = Add(x=w581, y=w565) -> (x+y=w567:i32)
                  n337 = Concatenate Strings("%0", w570, "d") -> (w573:string)
                  n338 = Format Into String(format string=w573, w567) -> (resulting string=w568:string)  [unwired: 2 in, 1 out]
                  n339 = Strip Path(path=w563) -> (stripped path=w564:path)  [unwired: 1 out]
                  n340 = Concatenate Strings(w580, w568, w575) -> (w578:string)
                  n341 = Build Path(base path=w564, name or relative path=w578) -> (appended path=w574:path)
                  n342 = call <vilib>:"Check if File or Folder Exists.vi"("path"=w574) -> ("error out"=w579:errorcluster, "file or folder exists?"=w577:bool, "dup path"=w576:path)  [unwired: 8 in]
                  n343 = call <vilib>:"Clear Errors.vi"("error in (no error)"=w579) -> ()  [unwired: 5 in, 2 out]
                  n344 = case shown="True" w577 {
                    frame False {
                    }
                    frame True {
                      n345 = Increment(x="Valid Scans") -> (x+1=w583:i32)
                      n346 = local write "Valid Scans"(w583) -> ()
                    }
                  }
                }
              }
              frame "Radio Selection 2" {
                n347 = local read "Data layout"() -> (w589:u16)
                n348 = stacked-sequence {
                  tunnel: w585 -> [w599 _]
                  tunnel: w590 -> [w598 w618]
                  tunnel: w591 -> [w597 w617]
                  tunnel: [w596 _] -> w586
                  tunnel: w589 -> [w595 _]
                  tunnel: [_ w618] -> w588
                  tunnel: [_ w617] -> w587
                  frame #0 {
                    n349 = case shown="1" w595 {
                      tunnel: w599 -> [w607 w616]
                      tunnel: w598 -> [w606 _]
                      tunnel: w597 -> [w604 w615]
                      tunnel: [w603 w614] -> w596
                      frame 0, Default {
                        n350 = call-poly <vilib>:"Read From Spreadsheet File.vi"("transpose (no:F)"=TRUE, "file path (dialog if empty)"=w607) -> ("all rows"=w612:dbl[][])  [unwired: 5 in, 4 out]
                        n351 = Delete From Array(array=w612, length=1, index (col)=0) -> (array with subset deleted=w609:dbl[][])  [unwired: 1 in, 1 out]
                        n352 = Array Size(array=w609) -> (size(s)=w608:i32[])
                        n353 = Index Array(array=w608) -> (element=w602:i32)  [unwired: 1 in]
                        n354 = Decrement(x=w602) -> (x-1=w601:i32)
                        n355 = Subtract(x=w601, y=w606) -> (x-y=w605:i32)
                        n356 = Divide(x=w605, y=w604) -> (x/y=w600:dbl)
                        n357 = Round Toward +Infinity(x=w600) -> (ceil(x): smallest int >= x=w603:dbl)
                      }
                      frame 1 {
                        n358 = call "DB HOR count.vi"("file path"=w616, "gap"=w615) -> ("number of scans"=w614:i32)  [unwired: 13 in]
                      }
                    }
                  }
                  frame #1 {
                  }
                }
                n359 = for {
                  N: w586 -> [_]
                  tunnel: w588 -> [w619]
                  tunnel: w587 -> [w621]
                  tunnel: [w623] -> w593 mode=indexing
                  i -> [w620]
                  n360 = Multiply(x=w621, y=w620) -> (x*y=w622:i32)
                  n361 = Add(x=w619, y=w622) -> (x+y=w623:i32)
                }
                n362 = Array Size(array=w593) -> (size(s)=w594:i32)
                n363 = local write "Valid Scans"(w594) -> ()
              }
            }
          }
          frame #1 {
            w638 = sgl[][] []
            n364 = local read "Crop bottom"() -> (w633:dbl)
            n365 = local read "Crop top"() -> (w634:i32)
            n366 = case shown="\"Radio Selection 2\"" w632 {
              tunnel: w634 -> [_ w661]
              tunnel: w633 -> [_ w660]
              tunnel: "Start wavelength" -> [_ w659]
              tunnel: "End wavelength" -> [_ w658]
              tunnel: w631 -> [_ w657]
              tunnel: [_ w654] -> w627
              tunnel: [_ w653] -> w626
              frame "Radio Selection 1", Default {
              }
              frame "Radio Selection 2" {
                n367 = local read "Data layout"() -> (w656:u16)
                n368 = local read "first file loc"() -> (w655:path)
                n369 = local read "Delimit"() -> (w652:string)
                n370 = case shown="0, Default" w656 {
                  tunnel: w661 -> [w670 _]
                  tunnel: w660 -> [w669 _]
                  tunnel: w659 -> [w668 _]
                  tunnel: w658 -> [w667 _]
                  tunnel: w657 -> [w666 _]
                  tunnel: [w665 _] -> w654
                  tunnel: [w664 _] -> w653
                  tunnel: w655 -> [w663 _]
                  tunnel: w652 -> [w662 _]
                  frame 0, Default {
                    n371 = call "Open scan DB.vi"("scan array"=w666, "End wavelength"=w667, "Crop bottom"=w669, "Start wavelength"=w668, "delim"=w662, "Crop top"=w670, "dup path"=w663) -> ("wavelengths"=w664:sgl[], "intensitites"=w665:sgl[][])  [unwired: 3 in]
                  }
                  frame 1 {
                  }
                }
              }
            }
            n372 = local read "Valid Scans"() -> (w637:i32)
            n373 = To Double Precision Float(number=w637) -> (double precision float=w645:dbl)
            n374 = property on="stop" class="Bool (strict)"("Visible"=TRUE) -> ()  [unwired: 2 in, 2 out]
            n375 = property on="Filtering Peaks" class="Bool (strict)"("Caption.Text"="Loading data") -> ()  [unwired: 2 in, 2 out]
            n376 = for "Peak detection and ordering" {
              N: w637 -> [w683]
              tunnel: "Start wavelength" -> [w692]
              tunnel: "End wavelength" -> [w681]
              tunnel: [w697] -> w635 mode=indexing
              tunnel: [w682] -> w636
              shift-right: [w696] -> w642
              shift-left: w638 -> [w693]
              tunnel: w644 -> [w680]
              shift-right: [w691] -> w641
              shift-left: w638 -> [w690]
              tunnel: [w689] -> w624 mode=indexing
              shift-right: [w686] -> w640
              shift-left: w638 -> [w687]
              shift-right: [w684] -> w639
              shift-left: w638 -> [w685]
              tunnel: w634 -> [w678]
              tunnel: w633 -> [w677]
              tunnel: w627 -> [w676]
              tunnel: w626 -> [w675]
              tunnel: w631 -> [w674]
              shift-right: [w672] -> _
              shift-left: 0 -> [w673]
              i -> [w671]
              n377 = Index Array(array=w680, index=w671) -> (element=w679:path)
              n378 = Wait (ms)(milliseconds to wait=1) -> ()  [unwired: 1 out]
              n379 = property on="Detecting Peaks" class="Bool (strict)"("Blinking"=TRUE) -> ()  [unwired: 2 in, 2 out]
              n380 = stacked-sequence {
                seq-local: [w700 _] -> [_ w843]
                seq-local: [w699 _] -> [_ w844]
                tunnel: w692 -> [w706 _]
                tunnel: w681 -> [w718 _]
                tunnel: [_ w840] -> w691
                tunnel: [_ w841] -> w696
                tunnel: [w700 _] -> w697
                tunnel: [w699 _] -> w682
                tunnel: w693 -> [_ w842]
                tunnel: w679 -> [w707 _]
                tunnel: w690 -> [_ w839]
                tunnel: w683 -> [_ w832]
                tunnel: [w719 _] -> w689
                tunnel: w687 -> [_ w825]
                tunnel: [_ w828] -> w686
                tunnel: w685 -> [_ w827]
                tunnel: [_ w826] -> w684
                tunnel: w678 -> [w717 _]
                tunnel: w677 -> [w716 _]
                tunnel: w676 -> [w714 _]
                tunnel: w675 -> [w715 _]
                tunnel: w671 -> [w705 w823]
                tunnel: w674 -> [w711 _]
                tunnel: w673 -> [w712 _]
                tunnel: [w698 _] -> w672
                frame #0 {
                  # "Here be dragons"
                  n381 = local read "Gap between files"() -> (w709:i32)
                  n382 = Index Array(array=w711, index=w705) -> (element=w710:i32)
                  n383 = local read "File style"() -> (w708:enum32{"Radio Selection 1", "Radio Selection 2"})
                  n384 = case shown="\"Scan for time stamp\", Default" "Type" {
                    tunnel: w707 -> [w780 _]
                    tunnel: [w775 w820] -> w719
                    tunnel: w711 -> [_ w822]
                    tunnel: w705 -> [_ w821]
                    frame "Scan for time stamp", Default {
                      n385 = call-poly <vilib>:"Read From Spreadsheet File.vi"("file path (dialog if empty)"=w780) -> ("all rows"=w778:string[][])  [unwired: 6 in, 4 out]
                      n386 = case shown="1" "Ring" {
                        tunnel: ["[0-9]+[:][0-9]+[:][0-9]+" "[0-9]+[ ][0-9]+[ ][0-9]+"] -> w772
                        frame 0, Default {
                        }
                        frame 1 {
                        }
                      }
                      n387 = Index Array(array=w778, index (col)=0) -> (element=w779:string[])  [unwired: 1 in]
                      n388 = for {
                        tunnel: w779 -> [w815] mode=indexing
                        tunnel: w772 -> [w814]
                        tunnel: [w809] -> w774
                        n389 = Match Pattern(string=w815, regular expression=w814) -> (match substring=w811:string, offset past match=w813:i32)  [unwired: 1 in, 2 out]
                        n390 = Less Than 0?(x=w813) -> (x < 0?=w812:bool)
                        n391 = feedback #1() -> (w809:string)  [unwired: 1 in]
                        n392 = case shown="False" w812 {
                          tunnel: w811 -> [w816 _]
                          tunnel: [w816 w817] -> w810
                          tunnel: w809 -> [_ w817]
                          frame False {
                          }
                          frame True {
                          }
                        }
                        n393 = feedback-in #1(w810) -> ()
                      }
                      n394 = case shown="\"Use time since first scan\"" "Output" {
                        tunnel: w774 -> [_ w785]
                        tunnel: [_ w784] -> w775
                        frame "Use raw time stamps", Default {
                        }
                        frame "Use time since first scan" {
                          n395 = Scan From String(format string="%d:%d:%d", input string=w785) -> (error out=w783:errorcluster, output 1=w791:i32, output 2=w790:i32, output 3=w789:i32)  [unwired: 5 in, 2 out]
                          n396 = call <vilib>:"Clear Errors.vi"("error in (no error)"=w783) -> ()  [unwired: 5 in, 2 out]
                          n397 = stacked-sequence {
                            seq-local: [w798 _ _] -> [_ _ w807]
                            seq-local: [_ w802 _] -> [_ _ w806]
                            tunnel: w791 -> [w801 _ _]
                            tunnel: w790 -> [_ w804 _]
                            tunnel: w789 -> [_ _ w808]
                            tunnel: [_ _ w805] -> w786
                            frame #0 {
                              w799 = 60
                              n398 = Multiply(x=w801, y=w799) -> (x*y=w800:i32)
                              n399 = Multiply(x=w800, y=w799) -> (x*y=w798:i32)
                            }
                            frame #1 {
                              n400 = Multiply(x=w804, y=60) -> (x*y=w802:i32)
                            }
                            frame #2 {
                              n401 = Compound Arithmetic op=ADD(w808, w807, w806) -> (w805:i32)
                            }
                          }
                          n402 = local read "Scan"() -> (w788:i32)
                          n403 = Equal To 0?(x=w788) -> (x = 0?=w787:bool)
                          n404 = case shown="False" w787 {
                            tunnel: w786 -> [_ w797]
                            tunnel: w786 -> [w795 _]
                            tunnel: [w793 0] -> w784
                            frame False {
                              n405 = local read "T0"() -> (w794:i32)
                              n406 = Subtract(x=w795, y=w794) -> (x-y=w793:i32)
                            }
                            frame True {
                              "T0" <- w797
                            }
                          }
                        }
                      }
                    }
                    frame "Manual scan frequency" {
                      n407 = Index Array(array=w822, index=w821) -> (element=w819:i32)
                      n408 = Multiply(x=w819, y="Numeric") -> (x*y=w820:i32)
                    }
                  }
                  n409 = case shown="\"Radio Selection 2\"" w708 {
                    tunnel: w717 -> [w741 w749]
                    tunnel: w716 -> [w740 w748]
                    tunnel: w707 -> [w739 _]
                    tunnel: w718 -> [w738 w747]
                    tunnel: [w734 w753] -> w704
                    tunnel: w706 -> [w737 w746]
                    tunnel: [w735 w750] -> w699
                    tunnel: w715 -> [_ w751]
                    tunnel: w714 -> [_ w755]
                    tunnel: w705 -> [_ w754]
                    tunnel: w712 -> [_ w745]
                    tunnel: [_ w744] -> w698
                    tunnel: w710 -> [_ w743]
                    tunnel: w709 -> [_ w742]
                    frame "Radio Selection 1", Default {
                      n410 = local read "Delimit"() -> (w736:string)
                      n411 = call "Open scan SEQ.vi"("dup path"=w739, "End wavelength"=w738, "Crop top"=w741, "delim"=w736, "Crop bottom"=w740, "Start wavelength"=w737) -> ("wavelengths"=w732:sgl[], "Intensities"=w733:sgl[])  [unwired: 8 in]
                      n412 = call "Crop Zero.vi"("Paired data"=w733, "Search data"=w732) -> ("Paired data out"=w734:sgl[], "Searched data out"=w735:sgl[])
                    }
                    frame "Radio Selection 2" {
                      n413 = local read "Data layout"() -> (w752:u16)
                      n414 = case shown="1" w752 {
                        tunnel: w755 -> [w759 _]
                        tunnel: w754 -> [w758 _]
                        tunnel: [w757 w760] -> w753
                        tunnel: w751 -> [w756 _]
                        tunnel: [w756 w762] -> w750
                        tunnel: w749 -> [_ w767]
                        tunnel: w748 -> [_ w770]
                        tunnel: w747 -> [_ w768]
                        tunnel: w746 -> [_ w769]
                        tunnel: w745 -> [_ w771]
                        tunnel: [_ w766] -> w744
                        tunnel: w743 -> [_ _]
                        tunnel: w742 -> [_ w764]
                        frame 0, Default {
                          n415 = Index Array(array=w759, index (row)=w758) -> (element=w757:sgl[])  [unwired: 1 in]
                        }
                        frame 1 {
                          n416 = local read "first file loc"() -> (w765:path)
                          n417 = call "Open scan DB HOR.vi"("dup path"=w765, "Bytes"=w771, "Crop top"=w767, "Crop bottom"=w770, "Start wavelength"=w769, "End wavelength"=w768, "gap"=w764) -> ("Bytes done"=w766:i64, "Intensity"=w761:sgl[], "wavelengths"=w763:sgl[])  [unwired: 6 in]
                          n418 = call "Crop Zero.vi"("Paired data"=w761, "Search data"=w763) -> ("Paired data out"=w760:sgl[], "Searched data out"=w762:sgl[])
                        }
                      }
                    }
                  }
                  n419 = case shown="True" "Norm" {
                    tunnel: w704 -> [w726 w728]
                    tunnel: [w726 w727] -> w701
                    frame False {
                    }
                    frame True {
                      n420 = Array Max & Min(array=w728) -> (max value=w731:sgl)  [unwired: 3 out]
                      n421 = Divide(x=100, y=w731) -> (x/y=w729:sgl)
                      n422 = Multiply(x=w729, y=w728) -> (x*y=w727:sgl[])
                    }
                  }
                  n423 = local read "Substract"() -> (w702:bool)
                  n424 = case shown="True" w702 {
                    tunnel: w701 -> [w720 w723]
                    tunnel: [w720 w722] -> w700
                    frame False {
                    }
                    frame True {
                      n425 = local read "subarray"() -> (w721:dbl[])
                      n426 = Divide(x=w723, y=w721) -> (x/y=w724:dbl[])
                      n427 = Multiply(x=w724, y=100) -> (x*y=w722:dbl[])
                    }
                  }
                }
                frame #1 {
                  n428 = Equal?(x=w832, y=w823) -> (x = y?=w831:bool)
                  n429 = Not(x="stop") -> (.not. x?=w830:bool)
                  n430 = And(x=w830, y="Vallys (T/F)") -> (x .and. y?=w829:bool)
                  n431 = And(x="Peaks (T/F)", y=w830) -> (x .and. y?=w836:bool)
                  n432 = case shown="True" w829 {
                    tunnel: w844 -> [_ w855]
                    tunnel: w843 -> [_ w854]
                    tunnel: w842 -> [w846 w866]
                    tunnel: [w846 w869] -> w841
                    tunnel: [w845 w868] -> w840
                    tunnel: w839 -> [w845 w847]
                    tunnel: "Minium length" -> [_ w865]
                    tunnel: "EnH choice" -> [_ w863]
                    tunnel: w831 -> [_ w848]
                    tunnel: "Poly order" -> [_ w849]
                    frame False {
                    }
                    frame True {
                      w873 = u16 1 items=["Peaks", "Valleys"] ("peaks/valleys")
                      n433 = while {
                        tunnel: "Lower \nthreshold" -> [w880]
                        shift-right: [w884] -> w851
                        shift-left: w854 -> [w878]
                        shift-right: [w881] -> w852
                        shift-left: w855 -> [w882]
                        stop <- w885 stop-if-true
                        n434 = Array Max & Min(array=w878) -> (min value=w879:dbl, min index (indices)=w883:i32)  [unwired: 2 out]
                        n435 = Greater Or Equal?(x=w879, y=w880) -> (x >= y?=w886:bool)
                        n436 = case shown="False" w886 {
                          tunnel: [FALSE TRUE] -> w885
                          tunnel: w878 -> [w891 w893]
                          tunnel: [w890 w893] -> w884
                          tunnel: w883 -> [w887 _]
                          tunnel: w882 -> [w889 w894]
                          tunnel: [w888 w894] -> w881
                          frame False {
                            n437 = Delete From Array(array=w889, index=w887) -> (array with subset deleted=w888:sgl[])  [unwired: 1 in, 1 out]
                            n438 = Delete From Array(array=w891, index=w887) -> (array with subset deleted=w890:dbl[])  [unwired: 1 in, 1 out]
                          }
                          frame True {
                          }
                        }
                      }
                      n439 = call-poly <vilib>:"Waveform Peak Detection.vi"("end of data (T)"=w848, "peaks/valleys"=w873, "width"="Width", "threshold"="Threshold", "Signal In"=w851) -> ("2nd Derivatives"=w859:dbl[], "Amplitudes"=w874:dbl[], "Locations"=w875:dbl[])  [unwired: 2 in, 2 out]
                      n440 = To Single Precision Float(number=w875) -> (single precision float=w861:sgl[])
                      n441 = To Single Precision Float(number=w874) -> (single precision float=w860:sgl[])
                      n442 = call "Pointyness screening.vi"("Scan Loc"=w852, "Feature Loc"=w861, "Intensities"=w860, "Peak\npointyness"="Vally\npointyness", "2nd Derivatives"=w859) -> ("Scan Loc"=w857:dbl[], "Feature Loc"=w856:dbl[], "Intensities"=w850:dbl[])  [unwired: 1 in]
                      n443 = call "feature locator.vi"("Features"=w856, "Locations"=w857) -> ("Feature locations"=w862:dbl[])
                      n444 = Build Array (concatenate)(w866, w862) -> (w870:dbl[][])
                      n445 = local read "Scan"() -> (w864:i32)
                      n446 = call "Peak tracking sq.vi"("BF len"=w865, "EnH choice"=w863, "Error control"="% tracking \nerror V", "Trace"=w864, "Poly count"=w849, "Int IN"=w850, "Scan"=w870) -> ("Int Out"=w871:sgl[], "Scan Out"=w872:sgl[])  [unwired: 3 in]
                      n447 = Build Array (concatenate)(w866, w872) -> (w869:sgl[][])
                      n448 = Build Array (concatenate)(w847, w871) -> (w868:sgl[][])
                    }
                  }
                  n449 = property on="stop" class="Bool (strict)"("Visible"=w830) -> ()  [unwired: 2 in, 2 out]
                  n450 = case shown="True" w836 {
                    tunnel: w844 -> [_ w915]
                    tunnel: w843 -> [_ w920]
                    tunnel: w825 -> [w897 w905]
                    tunnel: w827 -> [w896 w906]
                    tunnel: [w897 w904] -> w828
                    tunnel: [w896 w903] -> w826
                    tunnel: "EnH choice" -> [_ w917]
                    tunnel: "Minium length" -> [_ w918]
                    tunnel: w831 -> [_ w919]
                    tunnel: "Poly order" -> [_ w916]
                    frame False {
                    }
                    frame True {
                      w925 = u16 0 items=["Peaks", "Valleys"] ("peaks/valleys")
                      n451 = call-poly <vilib>:"Waveform Peak Detection.vi"("end of data (T)"=w919, "peaks/valleys"=w925, "width"="Width 2", "threshold"="Threshold  2", "Signal In"=w920) -> ("2nd Derivatives"=w911:dbl[], "Amplitudes"=w921:dbl[], "Locations"=w922:dbl[])  [unwired: 2 in, 2 out]
                      n452 = To Single Precision Float(number=w922) -> (single precision float=w914:sgl[])
                      n453 = To Single Precision Float(number=w921) -> (single precision float=w912:sgl[])
                      n454 = call "Pointyness screening.vi"("Scan Loc"=w915, "Feature Loc"=w914, "Intensities"=w912, "Peak\npointyness"="Peak\npointyness", "2nd Derivatives"=w911) -> ("Scan Loc"=w909:dbl[], "Feature Loc"=w913:dbl[], "Intensities"=w908:dbl[])  [unwired: 1 in]
                      n455 = call "feature locator.vi"("Features"=w913, "Locations"=w909) -> ("Feature locations"=w907:dbl[])
                      n456 = local read "Scan"() -> (w902:i32)
                      n457 = Build Array (concatenate)(w905, w907) -> (w900:dbl[][])
                      n458 = call "Peak tracking sq.vi"("BF len"=w918, "EnH choice"=w917, "Error control"="% tracking \nerror", "Trace"=w902, "Poly count"=w916, "Int IN"=w908, "Scan"=w900) -> ("Int Out"=w898:sgl[], "Scan Out"=w899:sgl[])  [unwired: 3 in]
                      n459 = Build Array (concatenate)(w905, w899) -> (w904:sgl[][])
                      n460 = Build Array (concatenate)(w906, w898) -> (w903:sgl[][])
                    }
                  }
                }
              }
              n461 = property on="Filtering Peaks" class="Bool (strict)"("Caption.Text"="Finding features...") -> ()  [unwired: 2 in, 2 out]
              "Scan" <- w671
            }
            "Croppped wave" <- w636
            "intensities" <- w635
            n462 = property on="Scan" class="Slide (strict)"("Scale.Maximum"=w645) -> ()  [unwired: 2 in, 2 out]
            n463 = case shown="True" "Save to file" {
              tunnel: w624 -> [_ w649]
              frame False {
              }
              frame True {
                n464 = call "File Dialog"() -> ("selected path"=w647:path, "cancelled"=w648:bool)  [unwired: 12 in, 2 out]
                n465 = case shown="False" w648 {
                  tunnel: w649 -> [w651 _]
                  tunnel: w647 -> [w650 _]
                  frame False {
                    n466 = call-poly <vilib>:"Write To Spreadsheet File.vi"("1D data"=w651, "file path (dialog if empty)"=w650) -> ()  [unwired: 6 in, 1 out]
                  }
                  frame True {
                  }
                }
              }
            }
          }
          frame #2 {
            w937 = FALSE
            w938 = TRUE
            n467 = in-place {
              n468 = in-place-match #2(w935) -> (w946:sgl[][])
              n469 = in-place-match #3(w934) -> (w945:sgl[][])
              n470 = in-place-match #4(w931) -> (w941:sgl[][])
              n471 = in-place-match #5(w930) -> (w942:sgl[][])
              n472 = stacked-sequence "Peak filter" {
                tunnel: w946 -> [w948 _]
                tunnel: w945 -> [w956 _]
                tunnel: [w955 _] -> w944
                tunnel: [w954 _] -> w943
                tunnel: [_ w985] -> w939
                tunnel: [_ w986] -> w940
                tunnel: w941 -> [_ w987]
                tunnel: w942 -> [_ w988]
                frame #0 {
                  n473 = Array Size(array=w948) -> (size(s)=w951:i32[])
                  n474 = Transpose 2D Array(2D array=w948) -> (transposed array=w953:sgl[][])
                  n475 = Index Array(array=w951, index=1) -> (element=w947:i32)
                  n476 = while {
                    tunnel: w953 -> [w959] mode=indexing
                    shift-right: [w970] -> w955
                    shift-left: w948 -> [w960]
                    shift-right: [w969] -> w954
                    shift-left: w956 -> [w962]
                    shift-right: [w966] -> _
                    shift-left: 0 -> [w965]
                    tunnel: w947 -> [w957]
                    i -> [w963]
                    stop <- w973 stop-if-true
                    n477 = call "Crop Zero.vi"("Search data"=w959) -> ("Searched data out"=w958:sgl[])  [unwired: 1 in, 1 out]
                    n478 = Add(x=w965, y=0) -> (x+y=w961:i32)
                    n479 = Equal?(x=w957, y=w963) -> (x = y?=w973:bool)
                    n480 = Array Size(array=w958) -> (size(s)=w972:i32)
                    n481 = local write "Scan"(w963) -> ()
                    n482 = Greater?(x=w972, y="Tracking \nTollerance P") -> (0:w971:bool)
                    n483 = case shown="False" w971 {
                      tunnel: w960 -> [w981 w984]
                      tunnel: [w980 w984] -> w970
                      tunnel: w962 -> [w979 w983]
                      tunnel: [w978 w983] -> w969
                      tunnel: [w977 w982] -> w967
                      tunnel: w961 -> [w974 w982]
                      frame False {
                        n484 = Delete From Array(array=w981, length=1, index (col)=w974) -> (array with subset deleted=w980:sgl[][])  [unwired: 1 in, 1 out]
                        n485 = Delete From Array(array=w979, length=1, index (col)=w974) -> (array with subset deleted=w978:sgl[][])  [unwired: 1 in, 1 out]
                        n486 = Decrement(x=w974) -> (x-1=w977:i32)
                      }
                      frame True {
                      }
                    }
                    n487 = Increment(x=w967) -> (x+1=w966:i32)
                  }
                  n488 = property on="Scan" class="Slide (strict)"("Scale.Maximum"=w947) -> ()  [unwired: 2 in, 2 out]
                  n489 = property on="Filtering Peaks" class="Bool (strict)"("Caption.Text"="Filtering peaks....") -> ()  [unwired: 2 in, 2 out]
                }
                frame #1 {
                  n490 = Array Size(array=w987) -> (size(s)=w992:i32[])
                  n491 = Transpose 2D Array(2D array=w987) -> (transposed array=w994:sgl[][])
                  n492 = Index Array(array=w992, index=1) -> (element=w989:i32)
                  n493 = while {
                    tunnel: w994 -> [w998] mode=indexing
                    shift-right: [w1008] -> w986
                    shift-left: w987 -> [w999]
                    shift-right: [w1007] -> w985
                    shift-left: w988 -> [w1001]
                    shift-right: [w1005] -> _
                    shift-left: 0 -> [w1004]
                    tunnel: w989 -> [w996]
                    i -> [w1002]
                    stop <- w1011 stop-if-true
                    n494 = call "Crop Zero.vi"("Search data"=w998) -> ("Searched data out"=w997:sgl[])  [unwired: 1 in, 1 out]
                    n495 = Add(x=w1004, y=0) -> (x+y=w1000:i32)
                    n496 = Equal?(x=w996, y=w1002) -> (x = y?=w1011:bool)
                    n497 = Array Size(array=w997) -> (size(s)=w1010:i32)
                    n498 = local write "Scan"(w1002) -> ()
                    n499 = Greater?(x=w1010, y="Tracking \nTollerance V") -> (0:w1009:bool)
                    n500 = case shown="False" w1009 {
                      tunnel: w999 -> [w1019 w1022]
                      tunnel: [w1018 w1022] -> w1008
                      tunnel: w1001 -> [w1017 w1021]
                      tunnel: [w1016 w1021] -> w1007
                      tunnel: [w1015 w1020] -> w1006
                      tunnel: w1000 -> [w1012 w1020]
                      frame False {
                        n501 = Delete From Array(array=w1019, length=1, index (col)=w1012) -> (array with subset deleted=w1018:sgl[][])  [unwired: 1 in, 1 out]
                        n502 = Delete From Array(array=w1017, length=1, index (col)=w1012) -> (array with subset deleted=w1016:sgl[][])  [unwired: 1 in, 1 out]
                        n503 = Decrement(x=w1012) -> (x-1=w1015:i32)
                      }
                      frame True {
                      }
                    }
                    n504 = Increment(x=w1006) -> (x+1=w1005:i32)
                  }
                  n505 = property on="Scan" class="Slide (strict)"("Scale.Maximum"=w989) -> ()  [unwired: 2 in, 2 out]
                  n506 = property on="Filtering Peaks" class="Bool (strict)"("Caption.Text"="Filtering peaks....") -> ()  [unwired: 2 in, 2 out]
                }
              }
              n507 = in-place-match #2(w944) -> (w932:sgl[][])
              n508 = in-place-match #3(w943) -> (w933:sgl[][])
              n509 = in-place-match #4(w940) -> (w929:sgl[][])
              n510 = in-place-match #5(w939) -> (w928:sgl[][])
            }
            n511 = property on="Filtering Peaks" class="Bool (strict)"("Blinking"=w938) -> ()  [unwired: 2 in, 2 out]
            n512 = local write "stop"(w937) -> ()
            n513 = property on="Detecting Peaks" class="Bool (strict)"("Blinking"=w937) -> ()  [unwired: 2 in, 2 out]
            n514 = property on="stop" class="Bool (strict)"("Visible"=w937) -> ()  [unwired: 2 in, 2 out]
            "Detecting Peaks" <- w938
          }
          frame #3 {
            w1032 = TRUE
            n515 = property on="Filtering Peaks" class="Bool (strict)"("Blinking"=FALSE) -> ()  [unwired: 2 in, 2 out]
            n516 = property on="Saving Data" class="Bool (strict)"("Blinking"=w1032) -> ()  [unwired: 2 in, 2 out]
            n517 = property on="Filtering Peaks" class="Bool (strict)"("Caption.Text"="Saving data...") -> ()  [unwired: 2 in, 2 out]
            n518 = stacked-sequence "Saving peak and vally data" {
              seq-local: [w1036 _ _ _ _ _] -> [_ w1043 w1051 w1066 w1073 _]
              tunnel: w1029 -> [_ w1044 _ _ _ _]
              tunnel: w1028 -> [_ _ w1053 _ _ _]
              tunnel: w1027 -> [_ _ _ w1067 _ _]
              tunnel: w1024 -> [_ _ _ _ w1076 _]
              tunnel: w1030 -> [_ w1041 w1056 w1065 w1074 _]
              frame #0 {
                n519 = local read "first file loc"() -> (w1035:path)
                n520 = Strip Path(path=w1035) -> (stripped path=w1034:path)  [unwired: 1 out]
                n521 = Build Path(base path=w1034, name or relative path="data") -> (appended path=w1037:path)
                n522 = Create Folder(path (use dialog)=w1037) -> (created path=w1036:path, error out=w1039:errorcluster)  [unwired: 2 in, 1 out]
                n523 = call <vilib>:"Clear Errors.vi"("error in (no error)"=w1039) -> ()  [unwired: 5 in, 2 out]
              }
              frame #1 {
                n524 = Transpose 2D Array(2D array=w1044) -> (transposed array=w1042:sgl[][])
                n525 = local write "Scan"(0) -> ()
                n526 = property on="Scan" class="Slide (strict)"("Scale.Maximum"=4) -> ()  [unwired: 2 in, 2 out]
                n527 = Build Path(base path=w1043, name or relative path="Peak_wavelengths.csv") -> (appended path=w1047:path)
                n528 = Build Array (concatenate)(w1041, w1042) -> (w1040:sgl[][])
                n529 = call-poly <vilib>:"Write To Spreadsheet File.vi"("delimiter (\\t)"=",", "transpose? (no:F)"=TRUE, "2D data"=w1040, "file path (dialog if empty)"=w1047) -> ()  [unwired: 4 in, 1 out]
              }
              frame #2 {
                n530 = Transpose 2D Array(2D array=w1053) -> (transposed array=w1054:sgl[][])
                n531 = local write "Scan"(1) -> ()
                n532 = Build Array (concatenate)(w1056, w1054) -> (w1055:sgl[][])
                n533 = Transpose 2D Array(2D array=w1055) -> (transposed array=w1052:sgl[][])
                n534 = Build Path(base path=w1051, name or relative path="Peak_intensities.csv") -> (appended path=w1059:path)
                n535 = call-poly <vilib>:"Write To Spreadsheet File.vi"("delimiter (\\t)"=",", "transpose? (no:F)"=FALSE, "append to file? (new file:F)"=FALSE, "2D data"=w1052, "file path (dialog if empty)"=w1059) -> ()  [unwired: 3 in, 1 out]
              }
              frame #3 {
                n536 = Transpose 2D Array(2D array=w1067) -> (transposed array=w1064:sgl[][])
                n537 = local write "Scan"(2) -> ()
                n538 = Build Array (concatenate)(w1065, w1064) -> (w1063:sgl[][])
                n539 = Build Path(base path=w1066, name or relative path="Valley_wavelengths.csv") -> (appended path=w1072:path)
                n540 = call-poly <vilib>:"Write To Spreadsheet File.vi"("delimiter (\\t)"=",", "transpose? (no:F)"=TRUE, "2D data"=w1063, "file path (dialog if empty)"=w1072) -> ()  [unwired: 4 in, 1 out]
              }
              frame #4 {
                n541 = Transpose 2D Array(2D array=w1076) -> (transposed array=w1077:sgl[][])
                n542 = local write "Scan"(3) -> ()
                n543 = Build Array (concatenate)(w1074, w1077) -> (w1078:sgl[][])
                n544 = Transpose 2D Array(2D array=w1078) -> (transposed array=w1075:sgl[][])
                n545 = Build Path(base path=w1073, name or relative path="Valley_intensities.csv") -> (appended path=w1082:path)
                n546 = call-poly <vilib>:"Write To Spreadsheet File.vi"("delimiter (\\t)"=",", "transpose? (no:F)"=FALSE, "append to file? (new file:F)"=FALSE, "2D data"=w1075, "file path (dialog if empty)"=w1082) -> ()  [unwired: 3 in, 1 out]
              }
              frame #5 {
                n547 = local write "Scan"(4) -> ()
              }
            }
            n548 = local write "mark"(i32[] [] ("mark")) -> ()
            "Filtering Peaks" <- w1032
          }
          frame #4 {
            n549 = Transpose 2D Array(2D array=w1102) -> (transposed array=w1105:sgl[][])
            n550 = Transpose 2D Array(2D array=w1103) -> (transposed array=w1104:sgl[][])
            n551 = stacked-sequence "Plotting graphs of peaks" {
              tunnel: w1105 -> [_ w1124 _ _ _ _]
              tunnel: w1100 -> [_ _ w1137 _ _ _]
              tunnel: w1104 -> [_ _ _ w1147 _ _]
              tunnel: w1101 -> [_ _ _ _ w1158 _]
              tunnel: w1089 -> [_ _ _ _ _ w1172]
              tunnel: w1093 -> [_ _ _ _ _ w1173]
              frame #0 {
                w1119 = TRUE
                n552 = local read "Start wavelength"() -> (w1114:dbl)
                n553 = local read "Start file number"() -> (w1117:i32)
                n554 = local read "End wavelength"() -> (w1113:dbl)
                n555 = local read "Valid Scans"() -> (w1116:i32)
                n556 = local write "Scan"(0) -> ()
                n557 = property on="Saving Data" class="Bool (strict)"("Blinking"=FALSE) -> ()  [unwired: 2 in, 2 out]
                n558 = Add(x=w1116, y=w1117) -> (x+y=w1118:i32)
                n559 = property on="Filtering Peaks" class="Bool (strict)"("Caption.Text"="Plotting graphs...") -> ()  [unwired: 2 in, 2 out]
                n560 = property on="Movie Plot" class="XYGraph (strict)"("XScale.Maximum"=w1113, "XScale.Minimum"=w1114) -> ()  [unwired: 2 in, 2 out]
                n561 = property on="Plotting graph" class="Bool (strict)"("Blinking"=w1119) -> ()  [unwired: 2 in, 2 out]
                n562 = property on="Scrollbar" class="Scroll (strict)"("DocMax"=w1118, "CoerceMax"=TRUE) -> ()  [unwired: 2 in, 2 out]
                n563 = call <vilib>:"Set Busy.vi"() -> ()  [unwired: 10 in, 2 out]
                "Saving Data" <- w1119
              }
              frame #1 {
                n564 = local write "Scan"(1) -> ()
                n565 = Index Array(array=w1124, index (col)=0) -> (element=w1125:sgl[])  [unwired: 1 in]
                n566 = Array Size(array=w1125) -> (size(s)=w1123:i32)
                "Number of\npeaks found" <- w1123
                n567 = for {
                  N: w1123 -> [_]
                  i -> [w1128]
                  n568 = local read "Start wavelength"() -> (w1130:dbl)
                  n569 = local read "End wavelength"() -> (w1129:dbl)
                  n570 = To Unsigned Long Integer(number=w1128) -> (unsigned 32bit integer=w1132:u32)
                  n571 = property on="Peak position vs Trace number" class="WFGraph (strict)"("YScale.Maximum"=w1129, "YScale.Minimum"=w1130, "Active Plot"=w1132, "Plot.Plot Interpolation"=u8 0, "Plot.Point Style"=u8 13) -> (error out=w1134:errorcluster)  [unwired: 2 in, 1 out]
                  n572 = call <vilib>:"Clear Errors.vi"("error in (no error)"=w1134) -> ()  [unwired: 5 in, 2 out]
                }
                "Peak position vs Trace number" <- w1124
              }
              frame #2 {
                n573 = Transpose 2D Array(2D array=w1137) -> (transposed array=→"Peak Intensity vs Trace number":sgl[][])
                n574 = Index Array(array=w1137, index (col)=0) -> (element=w1138:sgl[])  [unwired: 1 in]
                n575 = local write "Scan"(2) -> ()
                n576 = Array Size(array=w1138) -> (size(s)=w1135:i32)
                n577 = for {
                  N: w1135 -> [_]
                  i -> [w1141]
                  n578 = To Unsigned Long Integer(number=w1141) -> (unsigned 32bit integer=w1144:u32)
                  n579 = property on="Peak Intensity vs Trace number" class="WFGraph (strict)"("Active Plot"=w1144, "Plot.Plot Interpolation"=u8 0, "Plot.Point Style"=u8 13) -> (error out=w1145:errorcluster)  [unwired: 2 in, 1 out]
                  n580 = call <vilib>:"Clear Errors.vi"("error in (no error)"=w1145) -> ()  [unwired: 5 in, 2 out]
                }
              }
              frame #3 {
                n581 = Index Array(array=w1147, index (col)=0) -> (element=w1148:sgl[])  [unwired: 1 in]
                n582 = local write "Scan"(3) -> ()
                n583 = Array Size(array=w1148) -> (size(s)=w1146:i32)
                "Number of\nvallys found" <- w1146
                n584 = for {
                  N: w1146 -> [_]
                  i -> [w1151]
                  n585 = local read "Start wavelength"() -> (w1156:dbl)
                  n586 = local read "End wavelength"() -> (w1157:dbl)
                  n587 = To Unsigned Long Integer(number=w1151) -> (unsigned 32bit integer=w1152:u32)
                  n588 = property on="Vally position vs Trace number" class="WFGraph (strict)"("YScale.Maximum"=w1157, "YScale.Minimum"=w1156, "Active Plot"=w1152, "Plot.Plot Interpolation"=u8 0, "Plot.Point Style"=u8 13) -> (error out=w1154:errorcluster)  [unwired: 2 in, 1 out]
                  n589 = call <vilib>:"Clear Errors.vi"("error in (no error)"=w1154) -> ()  [unwired: 5 in, 2 out]
                }
                "Vally position vs Trace number" <- w1147
                "Vally pos" <- w1147
              }
              frame #4 {
                n590 = local write "Scan"(4) -> ()
                n591 = Index Array(array=w1158, index (col)=0) -> (element=w1160:sgl[])  [unwired: 1 in]
                n592 = Array Size(array=w1160) -> (size(s)=w1159:i32)
                n593 = for {
                  N: w1159 -> [_]
                  i -> [w1163]
                  n594 = To Unsigned Long Integer(number=w1163) -> (unsigned 32bit integer=w1167:u32)
                  n595 = property on="Vally Intensity vs Trace number" class="WFGraph (strict)"("Active Plot"=w1167, "Plot.Plot Interpolation"=u8 0, "Plot.Point Style"=u8 13) -> (error out=w1164:errorcluster)  [unwired: 2 in, 1 out]
                  n596 = call <vilib>:"Clear Errors.vi"("error in (no error)"=w1164) -> ()  [unwired: 5 in, 2 out]
                }
                "Vally Intensity vs Trace number" <- w1158
              }
              frame #5 {
                n597 = call "Xscale fudge.vi"("x array"=w1172, "intensity array in"=w1173) -> ("xscale maximum"=w1171:sgl, "xscale minimum"=w1170:sgl, "intensity array out"=w1169:dbl[][])
                n598 = Transpose 2D Array(2D array=w1169) -> (transposed array=→"Intensity Graph":dbl[][])
                n599 = property on="Intensity Graph" class="IntGraph (strict)"("XScale.Maximum"=w1171, "XScale.Minimum"=w1170) -> ()  [unwired: 2 in, 2 out]
              }
            }
            n600 = Delete From Array(array=w1093, length=1000, index (row)=100) -> (array with subset deleted=w1092:dbl[][])  [unwired: 1 in, 1 out]
            n601 = call "Search 1D Array for Nearest.vi"("desired element"="Cross location", "1D Array"=w1089) -> ("closest index"=w1088:i32, "closest element"=w1086:dbl)  [unwired: 8 in]
            n602 = Index Array(array=w1092, index (col)=w1088) -> (element=w1097:dbl[])  [unwired: 1 in]
            n603 = Index Array(array=w1097, index=0) -> (element=w1096:dbl)
            n604 = Divide(x=w1096, y=5) -> (x/y=w1095:dbl)
            n605 = Subtract(x=w1096, y=w1095) -> (x-y=w1094:dbl)
            n606 = for {
              tunnel: w1097 -> [w1108] mode=indexing
              tunnel: w1094 -> [w1109]
              i -> [w1106]
              n607 = Greater?(x=w1109, y=w1108) -> (0:w1107:bool)
              n608 = case shown="True" w1107 {
                tunnel: w1106 -> [_ w1112]
                frame False {
                }
                frame True {
                  n609 = local read "mark"() -> (w1110:i32[])
                  n610 = Build Array (concatenate)(w1110, w1112) -> (→"mark":i32[])
                }
              }
            }
          }
          frame #5 {
            n611 = disable-structure shown="Disabled" {
              disable-tunnel: w1174 -> [w1175 _]
              frame Disabled {
                n612 = local read "mark"() -> (w1179:i32[])
                n613 = Array Size(array=w1179) -> (size(s)=w1177:i32)
                n614 = Add Array Elements(numeric array=w1179) -> (sum=w1178:i32)
                n615 = Divide(x=w1178, y=w1177) -> (x/y=w1176:dbl)
                "Mark position" <- w1176
                n616 = property on="Intensity Graph" class="IntGraph (strict)"("Cursor.Cursor X"=w1175, "Cursor.Cursor Y"=w1176) -> ()  [unwired: 2 in, 2 out]
              }
              frame Enabled {
              }
            }
            n617 = property on="Intensity Graph" class="IntGraph (strict)" props=["Active Cursor"]() -> ()  [unwired: 2 in, 3 out]
          }
          frame #6 {
            n618 = local write "Scan"(4) -> ()
            n619 = call <vilib>:"Unset Busy.vi"() -> ()  [unwired: 11 in, 1 out]
            n620 = property on="Plotting graph" class="Bool (strict)"("Blinking"=FALSE) -> ()  [unwired: 2 in, 2 out]
            n621 = property on="Filtering Peaks" class="Bool (strict)"("Caption.Text"="Finished") -> ()  [unwired: 2 in, 2 out]
            "Plotting graph" <- TRUE
          }
        }
      }
      frame False {
      }
    }
  }
